vi "IFA300FrontPanel.vi"() -> ()   [LabVIEW 2011]
uses:
  subVIs/IFA300Command.ctl
  ADAM Client/Sub VIs/ADAM Controls/Remember_value_mode.ctl
  ADAM Client/Sub VIs/ADAM Controls/Update_scan_value.ctl
  Anemometry/Anemometry Sub Vis/Globals/Preference_global.vi
panel:
  in  "SquareWaveTest":bool
  out "CopytoChannels":string[](array[string])
  in  "ApplytoAll":bool
  in  "Cable Length":u8(slide)=1 max=1 step=1 scale=0.0..1.0
  in  "Overheat Setting":dbl(slide)=1.5 min=1.0 max=2.0 step=0.1 scale=1.0..2.0 scale format="%#.1f"
  in  "ModeArray":cluster{bool, "Enable":bool}[](array[cluster])
  in  "RunAll":bool caption="StopAll"
  in  "Reset IFA":bool
  out "Overheat (Running)":dbl format="%#.1f"
  in  "Port Name":string(combo)="COM4"
  out "Current Case":string="EndProgram"
  in  "EndProgram":bool
  in  "RunStandby":u8(knob) max=1 step=1 scale=0.0..1.0
  out "Standby":bool=TRUE
  out "Running":bool
  in  "Channel Selector":string(combo)="Channel 1"
  in  "Offset":dbl min=0.0 max=10.24 step=0.5 format="%#.2g"
  in  "Gain":string(combo)="1\r\n"
  in  "Low-Pass Filter":string(combo)="None"
  in  "High-Pass Filter":string(combo)="None"
  in  "High Power Bridge":u8(slide) max=1 step=1 scale=0.0..1.0
  in  "Probe Type Selector":u8(slide)=1 max=2 step=1 scale=0.0..2.0
  out "Temperature":dbl
  in  "StopAll":bool
  out "TimeColdResRead":string
  out "TimeColdResMeas":string
  out "TimeCableResRead":string
  out "TimeCableResMeas":string caption="Date/Time"
  in  "ReadColdRes":bool
  in  "ReadCableRes":bool
  in  "MeasColdRes":bool
  in  "MeasCableRes":bool
  out "Hot Resistance":dbl format="%#.2f"
  out "Probe Resistance":dbl format="%#.2f"
  out "Cable Resistance":dbl format="%#.2f"
  # "CH1"
  # "CH2"
  # "CH3"
  # "CH4"
  # "CH5"
  # "CH6"
  # "CH7"
  # "CH8"
  # "Running"
  # "Enabled"
  # "Disabled"
  # "Standby"
  # "Run"
  # "30m"
  # "5m"
  # "On"
  # "Off"
  # "Wire"
  # "Film"
  # "Non-Cylindrical"
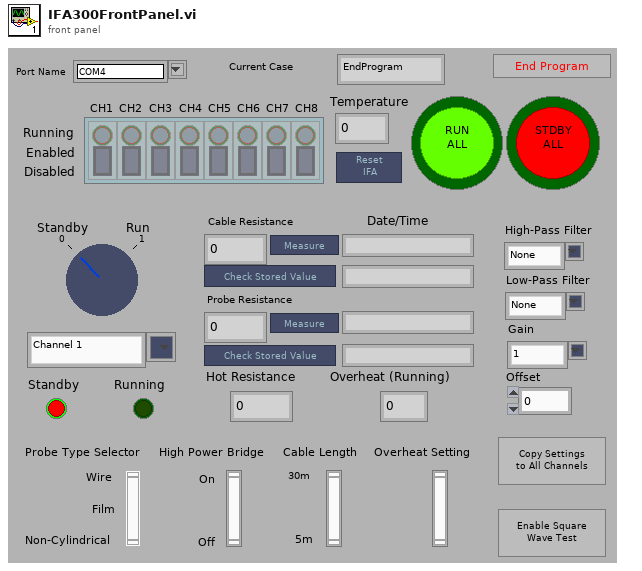
[diagram p1: front panel]
types:
  T1 = typedef "IFA300Command.ctl" = string
  T2 = typedef "Remember_value_mode.ctl" = enum16{"Read only", "Read and Write"}
  T3 = typedef "Update_scan_value.ctl" = cluster{"Channel Name":string, "New Value":dbl}
  T4 = cluster{"Running/Standby":string, "Enabled/Dissabled":string, "SecSince1904":string, "Date/TimeFileWritten":string}
  T5 = cluster{"Channel Selector":string, "RunAll":bool, "StopAll":bool, "EndProgram":bool, "MeasCableRes":bool, "ReadCableRes":bool, "MeasColdRes":bool, "ReadColdRes":bool, "Overheat Setting":dbl, "High-Pass Filter":string, "Low-Pass Filter":string, "Gain":string, "Offset":dbl, "RunStandby":u8, "Probe Type Selector":u8, "High Power Bridge":u8, "Cable Length":u8, "Reset IFA":bool, "ApplytoAll":bool, "SquareWaveTest":bool}
  T6 = cluster{"Channel Selector":bool, "RunAll":bool, "StopAll":bool, "EndProgram":bool, "MeasCableRes":bool, "ReadCableRes":bool, "MeasColdRes":bool, "ReadColdRes":bool, "Overheat Setting":bool, "High-Pass Filter":bool, "Low-Pass Filter":bool, "Gain":bool, "Offset":bool, "RunStandby":bool, "Probe Type Selector":bool, "High Power Bridge":bool, "Cable Length":bool, "Reset IFA":bool, "ApplytoAll":bool, "SquareWaveTest":bool}
  T7 = cluster{"Temperature":dbl, "Running":bool, "Standby":bool, "Cable Resistance":dbl, "Probe Resistance":dbl, "Hot Resistance":dbl, "Overheat (Running)":dbl, "Port Name":string, "TimeCableResMeas":string, "TimeCableResRead":string, "TimeColdResMeas":string, "TimeColdResRead":string}
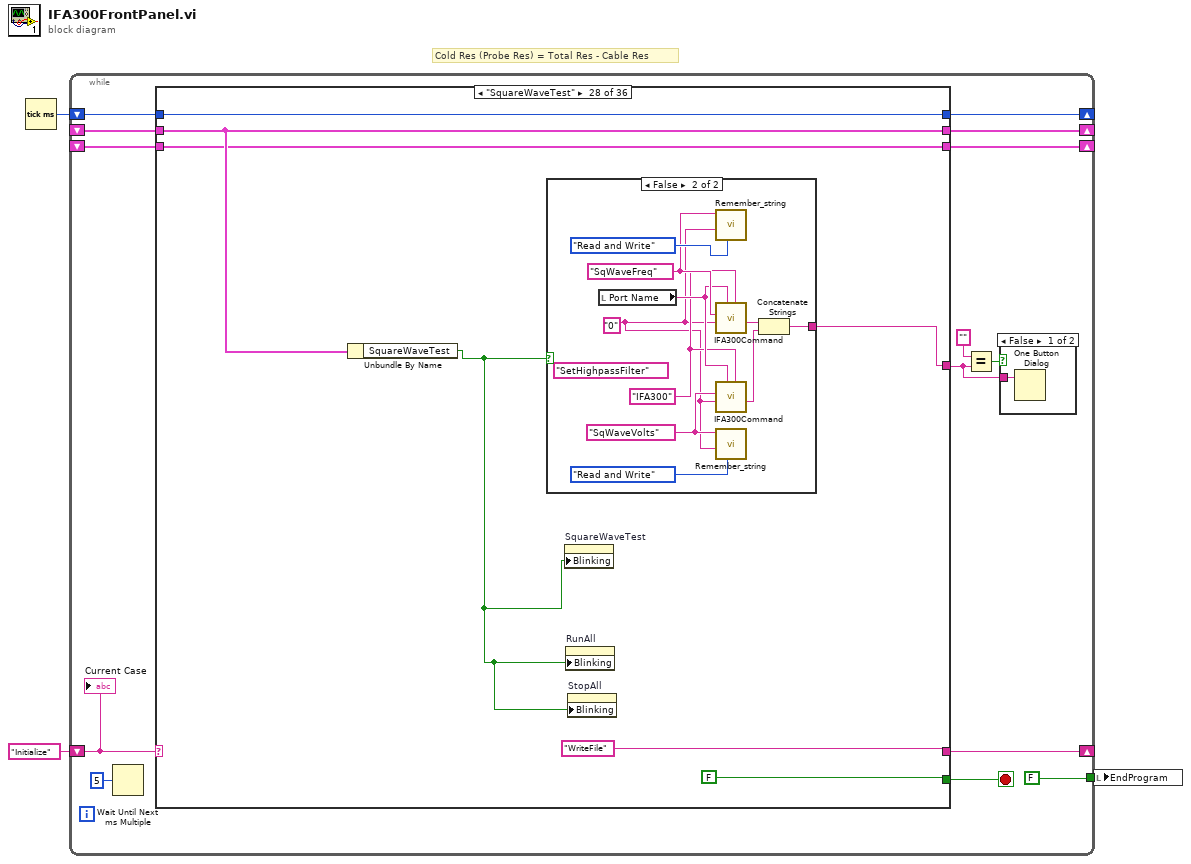
[diagram p0: block diagram]
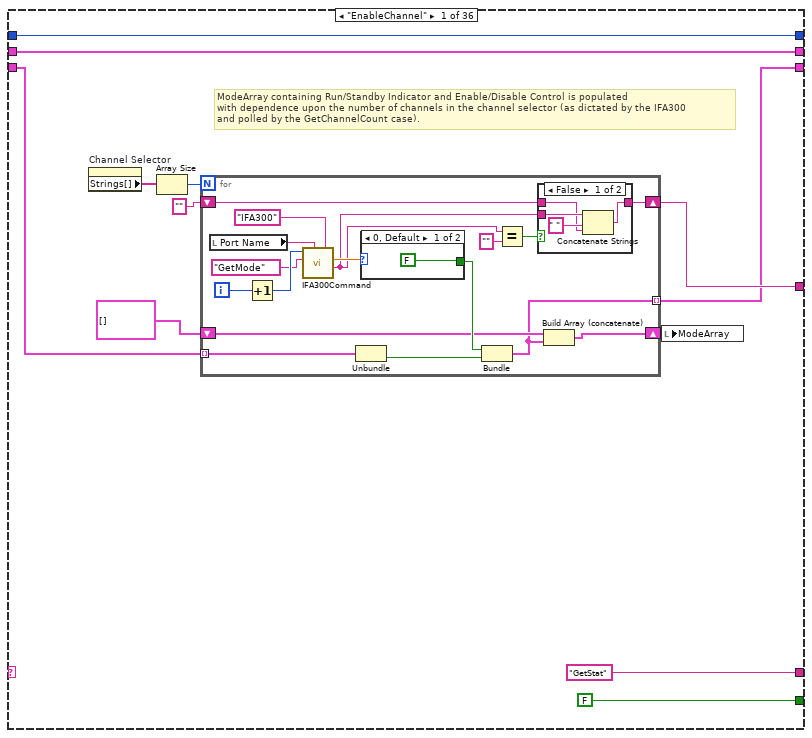
[diagram p3: hidden frame]
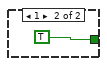
[diagram p5: hidden frame]
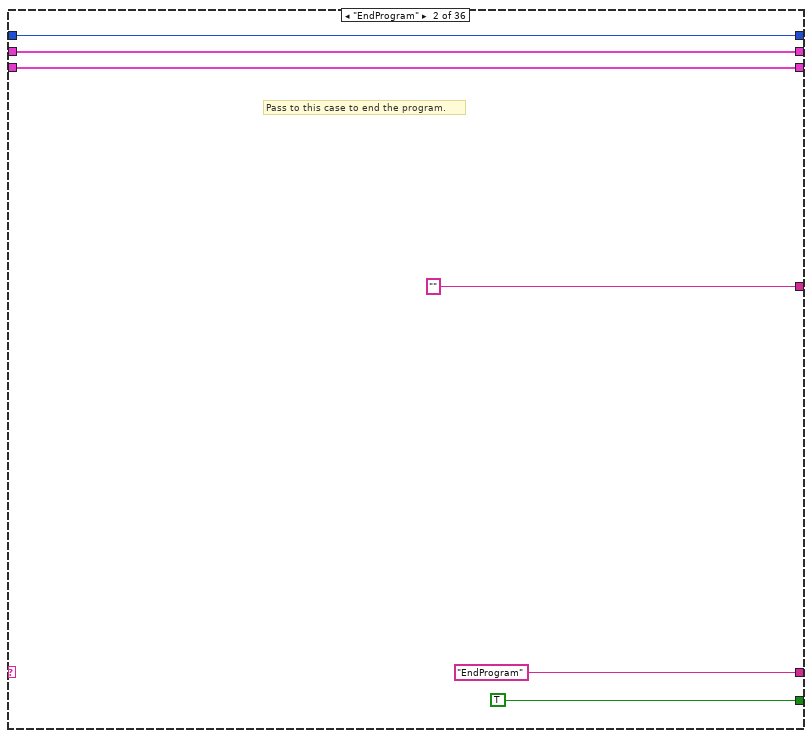
[diagram p6: hidden frame]
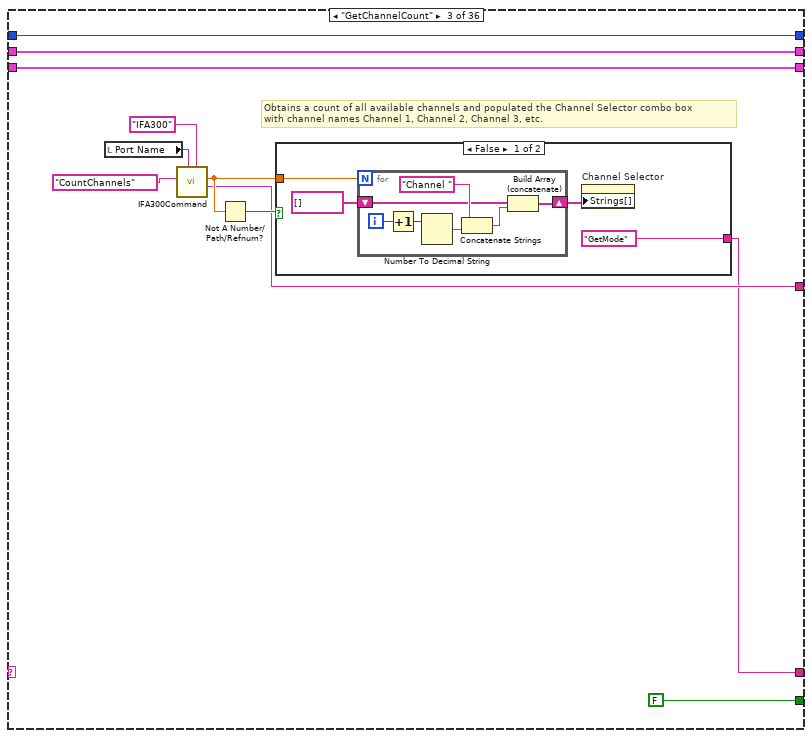
[diagram p7: hidden frame]
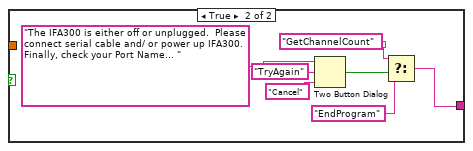
[diagram p8: hidden frame]
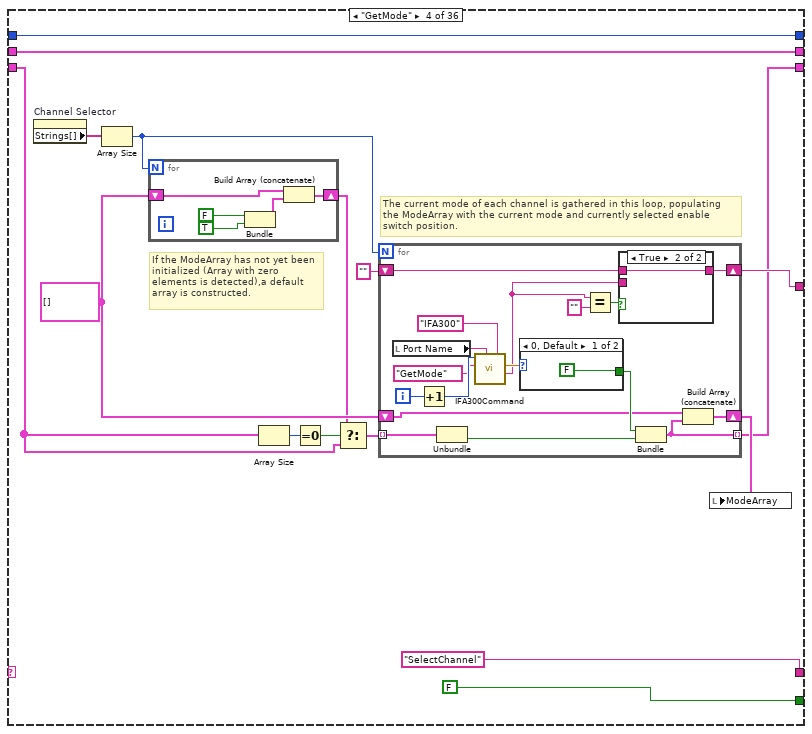
[diagram p9: hidden frame]
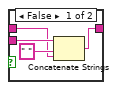
[diagram p10: hidden frame]
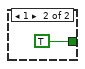
[diagram p11: hidden frame]
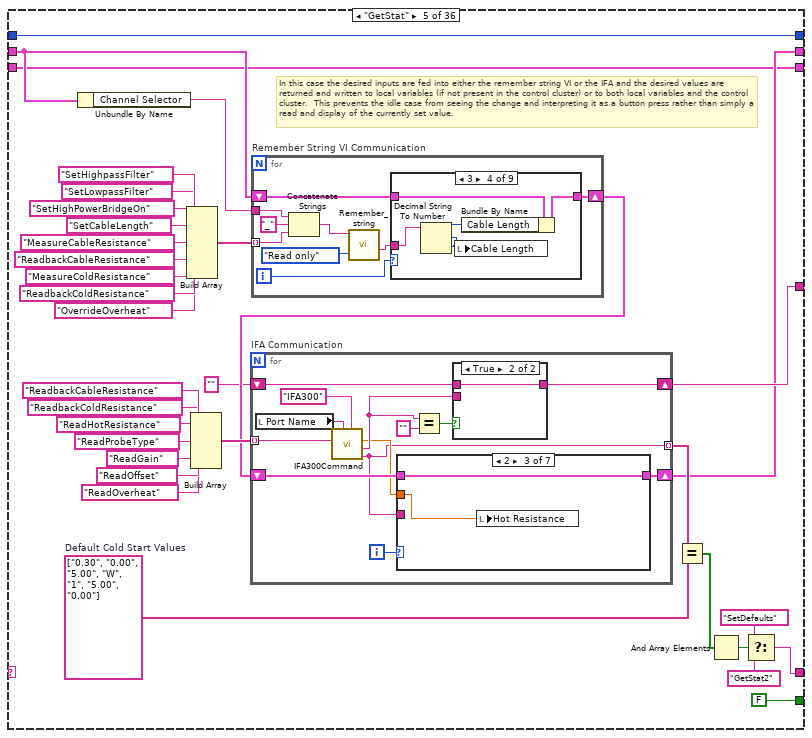
[diagram p12: hidden frame]
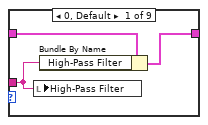
[diagram p13: hidden frame]
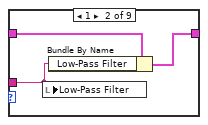
[diagram p14: hidden frame]
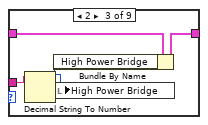
[diagram p15: hidden frame]
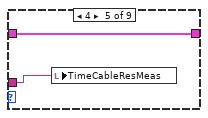
[diagram p16: hidden frame]
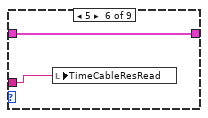
[diagram p17: hidden frame]
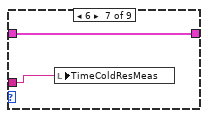
[diagram p18: hidden frame]
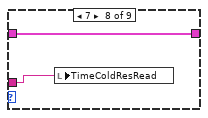
[diagram p19: hidden frame]
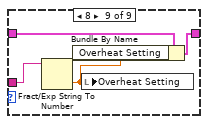
[diagram p20: hidden frame]
diagram:
  # "Cold Res (Probe Res) = Total Res - Cable Res"
  n1 = Tick Count (ms)() -> (millisecond timer value=w1:u32)
  n2 = while {
    shift-right: [w16] -> _
    shift-left: _ -> [w17]
    shift-right: [w14] -> _
    shift-left: "Initialize" -> [w12]
    tunnel: [FALSE ("EndProgram")] -> w2
    shift-right: [w6] -> _
    shift-left: w1 -> [w7]
    shift-right: [w5] -> _
    shift-left: _ -> [w4]
    stop <- w13 stop-if-true
    n3 = Wait Until Next ms Multiple(millisecond multiple=u32 5) -> ()  [unwired: 1 out]
    n4 = case shown="\"SquareWaveTest\"" w12 {
      tunnel: w17 -> [w28 w60 w64 w105 w145 w250 w290 w314 w371 _ w443 w464 w478 w486 w502 w533 w556 w573 w584 w598 w617 w624 w660 w685 w715 w795 w820 w835 w875 w905 w932 w967 w998 w1020 w1037 w1045]
      tunnel: [w28 w60 w64 w105 w137 w251 w290 w299 w375 w420 w443 w464 w478 w486 w502 w533 w556 w573 w584 w598 w617 w624 w660 w685 w716 w795 w820 w835 w875 w905 w932 w967 w998 w1020 w1037 w1071] -> w16
      tunnel: [FALSE ("EndProgram") TRUE ("EndProgram") FALSE ("EndProgram") FALSE ("EndProgram") FALSE ("EndProgram") FALSE ("EndProgram") FALSE ("EndProgram") FALSE ("EndProgram") FALSE ("EndProgram") FALSE ("EndProgram") FALSE ("EndProgram") FALSE ("EndProgram") FALSE ("EndProgram") TRUE ("EndProgram") FALSE ("EndProgram") FALSE ("EndProgram") FALSE ("EndProgram") FALSE ("EndProgram") FALSE ("EndProgram") FALSE ("EndProgram") FALSE ("EndProgram") FALSE ("EndProgram") FALSE ("EndProgram") FALSE ("EndProgram") FALSE ("EndProgram") FALSE ("EndProgram") FALSE ("EndProgram") FALSE ("EndProgram") FALSE ("EndProgram") FALSE ("EndProgram") FALSE ("EndProgram") FALSE ("EndProgram") FALSE ("EndProgram") FALSE ("EndProgram") FALSE ("EndProgram") FALSE ("EndProgram")] -> w13
      tunnel: ["GetStat" "EndProgram" w61 "SelectChannel" w155 "WriteFile" w272 w333 "SetProbeType" ("t") "GetChannelCount" "ReadCableRes" "ReadColdRes" "ReadTemperature" ("t") "NoMatch" w488 w523 "WriteFile" "WriteFile" "WriteFile" "Idle" ("t") "WriteFile" "GetMode" "GetStat" w668 "GetStat" ("t") w781 w802 "WriteFile" "ReadHotRes" w886 "GetMode" w956 w982 w1013 "GetMode" w1048] -> w14
      tunnel: [w21 "" ("Error Description") w65 w101 w161 w252 w289 "" ("Error Description") "" ("Error Description") "" ("x") w439 w462 w473 "" ("Error Description") w500 w522 w551 w565 w578 w600 w613 w622 w657 w680 w720 w793 w821 w831 w859 w901 w921 "" ("Error Description") w996 w1018 w1033 "" ("Error Description")] -> w8
      tunnel: w7 -> [w27 w56 w63 w99 w152 w259 w288 w335 w377 w402 w435 w458 _ w482 w498 w530 w549 w563 w577 w599 w612 w623 w656 w679 w717 w792 w812 w834 w863 w896 w926 w969 w995 w1017 w1031 w1080]
      tunnel: [w27 w56 w63 w99 w152 w259 w288 w335 w377 w402 w435 w458 w477 w482 w498 w530 w549 w563 w577 w599 w612 w623 w656 w679 w717 w792 w812 w834 w863 w896 w926 w969 w995 w1017 w1031 w1080] -> w6
      tunnel: [w19 w55 w62 w90 w136 w247 w277 w305 w376 "ModeArray" w426 w449 w472 w481 w487 w517 w548 w562 w576 w597 w606 w621 w655 w672 w714 w791 w806 w833 w858 w890 w914 w968 w994 w1016 w1030 w1077] -> w5
      tunnel: w4 -> [w20 w55 w62 w91 w136 w247 w277 w301 w376 _ w426 w449 w472 w481 w487 w517 w548 w562 w576 w597 w606 w621 w655 w672 w714 w791 w806 w833 w858 w890 w914 w968 w994 w1016 w1030 w1077]
      frame "EnableChannel" {
        # "ModeArray containing Run/Standby Indicator and Enable/Disable Control is populated\nwith dependence upon the number of channels in the channel selector (as dictated by the IFA300\nand polled by the GetChannelCount case)."
        n5 = property on="Channel Selector" class="CmbBox"() -> ("Strings[]"=w26:string[])  [unwired: 2 in, 2 out]
        n6 = Array Size(array=w26) -> (size(s)=w25:i32)
        n7 = for {
          N: w25 -> [_]
          shift-right: [w41] -> w21
          shift-left: "" -> [w40]
          shift-right: [w35] -> w22
          shift-left: cluster{bool, bool}[] [] -> [w34]
          tunnel: w20 -> [w33] mode=indexing
          tunnel: [w31] -> w19 mode=indexing
          i -> [w44]
          n8 = local read "Port Name"() -> (w46:string)
          n9 = Increment(x=w44) -> (x+1=w43:i32)
          n10 = call "IFA300Command.vi"("Channel Name"="IFA300", "Port Name"=w46, "IFACommand"=T1 "GetMode" ("IFA300Command"), "Address"=w43) -> ("Error Description"=w39:string, "Numeric Reply"=w45:dbl)  [unwired: 1 in, 4 out]
          n11 = Unbundle(w33) -> ("Enable"=w32:bool)  [unwired: 1 out]
          n12 = case shown="0, Default" w45 {
            tunnel: [FALSE TRUE] -> w36
            frame 0, Default {
            }
            frame 1 {
            }
          }
          n13 = Bundle(w36, "Enable"=w32) -> (w31:cluster{bool, "Enable":bool})  [unwired: 1 out]
          n14 = Equal?(x=w39, y="") -> (x = y?=w37:bool)
          n15 = case shown="False" w37 {
            tunnel: w39 -> [w50 _]
            tunnel: [w49 w52] -> w41
            tunnel: w40 -> [w48 w52]
            frame False {
              n16 = Concatenate Strings(w50, " " ("string"), w48) -> (w49:string)
            }
            frame True {
            }
          }
          n17 = Build Array (concatenate)(w34, w31) -> (w35:cluster{bool, "Enable":bool}[])
        }
        n18 = local write "ModeArray"(w22) -> ()
      }
      frame "EndProgram" {
        # "Pass to this case to end the program."
      }
      frame "GetChannelCount" {
        # "Obtains a count of all available channels and populated the Channel Selector combo box\nwith channel names Channel 1, Channel 2, Channel 3, etc."
        n19 = local read "Port Name"() -> (w69:string)
        n20 = call "IFA300Command.vi"("Channel Name"="IFA300", "Port Name"=w69, "IFACommand"=T1 "CountChannels" ("IFA300Command")) -> ("Error Description"=w65:string, "Numeric Reply"=w67:dbl)  [unwired: 2 in, 4 out]
        n21 = Not A Number/Path/Refnum?(number/path/refnum=w67) -> (NaN/Path/Refnum?=w66:bool)
        n22 = case shown="False" w66 {
          tunnel: w67 -> [w73 _]
          tunnel: ["GetMode" w84] -> w61
          frame False {
            n23 = for {
              N: w73 -> [_]
              shift-right: [w77] -> w74
              shift-left: string[] [] -> [w78]
              i -> [w81]
              n24 = Increment(x=w81) -> (x+1=w80:i32)
              n25 = Number To Decimal String(number=w80) -> (decimal integer string=w79:string)  [unwired: 1 out]
              n26 = Concatenate Strings("Channel ", w79) -> (w76:string)
              n27 = Build Array (concatenate)(w78, w76) -> (w77:string[])
            }
            n28 = property on="Channel Selector" class="CmbBox"("Strings[]"=w74) -> ()  [unwired: 2 in, 2 out]
          }
          frame True {
            n29 = Two Button Dialog(message="The IFA300 is either off or unplugged.  Please connect serial cable and/ or power up IFA300.  Finally, check your Port Name... ", 1:"Cancel" ("F button name (\"Cancel\")"), 2:"TryAgain" ("T button name (\"OK\")")) -> (T button?=w86:bool)
            n30 = Select(t="GetChannelCount", s=w86, f="EndProgram" ("t")) -> (s? t:f=w84:string)
          }
        }
      }
      frame "GetMode" {
        w93 = cluster{bool, bool}[] []
        # "The current mode of each channel is gathered in this loop, populating the ModeArray with the current mode and currently selected enable switch position."
        # "If the ModeArray has not yet been initialized (Array with zero elements is detected),a default array is constructed."
        n31 = property on="Channel Selector" class="CmbBox"() -> ("Strings[]"=w102:string[])  [unwired: 2 in, 2 out]
        n32 = Array Size(array=w102) -> (size(s)=w96:i32)
        n33 = for {
          N: w96 -> [_]
          shift-right: [w109] -> w92
          shift-left: w93 -> [w110]
          n34 = Bundle(FALSE, TRUE) -> (w108:cluster{bool, bool})  [unwired: 1 out]
          n35 = Build Array (concatenate)(w110, w108) -> (w109:cluster{bool, bool}[])
        }
        n36 = Array Size(array=w91) -> (size(s)=w97:i32)
        n37 = Equal To 0?(x=w97) -> (x = 0?=w95:bool)
        n38 = Select(t=w92, s=w95, f=w91) -> (s? t:f=w94:cluster{bool, "Enable":bool}[])
        n39 = for {
          N: w96 -> [_]
          shift-right: [w121] -> w101
          shift-left: "" -> [w120]
          shift-right: [w115] -> w98
          shift-left: w93 -> [w114]
          tunnel: w94 -> [w113] mode=indexing
          tunnel: [w111] -> w90 mode=indexing
          i -> [w124]
          n40 = local read "Port Name"() -> (w126:string)
          n41 = Increment(x=w124) -> (x+1=w123:i32)
          n42 = Unbundle(w113) -> ("Enable"=w112:bool)  [unwired: 1 out]
          n43 = call "IFA300Command.vi"("Channel Name"="IFA300", "Port Name"=w126, "IFACommand"=T1 "GetMode" ("IFA300Command"), "Address"=w123) -> ("Error Description"=w119:string, "Numeric Reply"=w125:dbl)  [unwired: 1 in, 4 out]
          n44 = case shown="0, Default" w125 {
            tunnel: [FALSE TRUE] -> w116
            frame 0, Default {
            }
            frame 1 {
            }
          }
          n45 = Equal?(x=w119, y="") -> (x = y?=w117:bool)
          n46 = case shown="True" w117 {
            tunnel: w119 -> [w130 _]
            tunnel: [w129 w132] -> w121
            tunnel: w120 -> [w128 w132]
            frame False {
              n47 = Concatenate Strings(w130, " " ("string"), w128) -> (w129:string)
            }
            frame True {
            }
          }
          n48 = Bundle(w116, "Enable"=w112) -> (w111:cluster{bool, "Enable":bool})  [unwired: 1 out]
          n49 = Build Array (concatenate)(w114, w111) -> (w115:cluster{bool, "Enable":bool}[])
        }
        n50 = local write "ModeArray"(w98) -> ()
      }
      frame "GetStat" {
        w159 = string[] ["0.30", "0.00", "5.00", "W", "1", "5.00", "0.00"]  # Default Cold Start Values
        # "In this case the desired inputs are fed into either the remember string VI or the IFA and the desired values are returned and written to local variables (if not present in the control cluster) or to both local variables and the control cluster.  This prevents the idle case from seeing the change and interpreting it as a button press rather than simply a read and display of the currently set value."
        n51 = Unbundle By Name(w145) -> ("Channel Selector"=w143:string)
        n52 = Build Array(T1 "SetHighpassFilter" ("IFA300Command"), T1 "SetLowpassFilter" ("IFA300Command"), T1 "SetHighPowerBridgeOn" ("IFA300Command"), T1 "SetCableLength" ("IFA300Command"), T1 "MeasureCableResistance" ("IFA300Command"), T1 "ReadbackCableResistance" ("IFA300Command"), T1 "MeasureColdResistance" ("IFA300Command"), T1 "ReadbackColdResistance" ("IFA300Command"), T1 "OverrideOverheat" ("element")) -> (w146:T1[])
        n53 = Build Array(T1 "ReadbackCableResistance" ("IFA300Command"), T1 "ReadbackColdResistance" ("IFA300Command"), T1 "ReadHotResistance" ("IFA300Command"), T1 "ReadProbeType" ("IFA300Command"), T1 "ReadGain" ("IFA300Command"), T1 "ReadOffset" ("IFA300Command"), T1 "ReadOverheat" ("IFA300Command")) -> (w160:T1[])
        n54 = for "Remember String VI Communication" {
          tunnel: w146 -> [w175] mode=indexing
          tunnel: w143 -> [w177]
          shift-right: [w169] -> w144
          shift-left: w145 -> [w170]
          i -> [w172]
          n55 = Concatenate Strings(w177, "_" ("string"), w175) -> (w174:string)
          n56 = call "Remember_string.vi"("Mode"=Remember_value_mode."Read only", "Ch name"=w174) -> ("Output Value"=w171:string)  [unwired: 2 in, 7 out]
          n57 = case shown="3" w172 {
            tunnel: w171 -> [w178 w181 w185 w189 w192 w194 w196 w198 w203]
            tunnel: w170 -> [w180 w183 w187 w191 w193 w195 w197 w199 w202]
            tunnel: [w179 w182 w186 w190 w193 w195 w197 w199 w201] -> w169
            frame 0, Default {
              n58 = local write "High-Pass Filter"(w178) -> ()
              n59 = Bundle By Name(cluster=w180, "High-Pass Filter"=w178) -> (w179:T5)
            }
            frame 1 {
              n60 = local write "Low-Pass Filter"(w181) -> ()
              n61 = Bundle By Name(cluster=w183, "Low-Pass Filter"=w181) -> (w182:T5)
            }
            frame 2 {
              n62 = Decimal String To Number(string=w185) -> (number=w184:i32)  [unwired: 3 out]
              n63 = Bundle By Name(cluster=w187, "High Power Bridge"=w184) -> (w186:T5)
              n64 = local write "High Power Bridge"(w184) -> ()
            }
            frame 3 {
              n65 = Decimal String To Number(string=w189) -> (number=w188:i32)  [unwired: 3 out]
              n66 = local write "Cable Length"(w188) -> ()
              n67 = Bundle By Name(cluster=w191, "Cable Length"=w188) -> (w190:T5)
            }
            frame 4 {
              n68 = local write "TimeCableResMeas"(w192) -> ()
            }
            frame 5 {
              n69 = local write "TimeCableResRead"(w194) -> ()
            }
            frame 6 {
              n70 = local write "TimeColdResMeas"(w196) -> ()
            }
            frame 7 {
              n71 = local write "TimeColdResRead"(w198) -> ()
            }
            frame 8 {
              n72 = Fract/Exp String To Number(string=w203) -> (number=w200:dbl)  [unwired: 4 out]
              n73 = Bundle By Name(cluster=w202, "Overheat Setting"=w200) -> (w201:T5)
              n74 = local write "Overheat Setting"(w200) -> ()
            }
          }
        }
        n75 = for "IFA Communication" {
          tunnel: w160 -> [w214] mode=indexing
          shift-right: [w211] -> w161
          shift-left: "" -> [w210]
          shift-right: [w205] -> w137
          shift-left: w144 -> [w207]
          tunnel: [w204] -> w151 mode=indexing
          i -> [w208]
          n76 = local read "Port Name"() -> (w215:string)
          n77 = call "IFA300Command.vi"("Channel Name"="IFA300", "Port Name"=w215, "IFACommand"=w214) -> ("String Reply"=w204:string, "Error Description"=w209:string, "Numeric Reply"=w206:dbl)  [unwired: 2 in, 3 out]
          n78 = case shown="2" w208 {
            tunnel: w207 -> [w218 w220 w222 w225 w232 w235 w236]
            tunnel: w204 -> [_ _ _ w224 w230 _ _]
            tunnel: w206 -> [w217 w219 w221 _ _ w233 w237]
            tunnel: [w218 w220 w222 w226 w231 w234 w236] -> w205
            frame 0, Default {
              n79 = local write "Cable Resistance"(w217) -> ()
            }
            frame 1 {
              n80 = local write "Probe Resistance"(w219) -> ()
            }
            frame 2 {
              n81 = local write "Hot Resistance"(w221) -> ()
            }
            frame 3 {
              n82 = case shown="\"F\", Default" w224 {
                tunnel: [u8 1 ("W/F/N Selector") u8 0 ("W/F/N Selector") u8 2 ("W/F/N Selector")] -> w223
                frame "F", Default {
                }
                frame "N" {
                }
                frame "W" {
                }
              }
              n83 = Bundle By Name(cluster=w225, "Probe Type Selector"=w223) -> (w226:T5)
              n84 = local write "Probe Type Selector"(w223) -> ()
            }
            frame 4 {
              n85 = local write "Gain"(w230) -> ()
              n86 = Bundle By Name(cluster=w232, "Gain"=w230) -> (w231:T5)
            }
            frame 5 {
              n87 = local write "Offset"(w233) -> ()
              n88 = Bundle By Name(cluster=w235, "Offset"=w233) -> (w234:T5)
            }
            frame 6 {
              n89 = local write "Overheat (Running)"(w237) -> ()
            }
          }
          n90 = Equal?(x=w209, y="") -> (x = y?=w213:bool)
          n91 = case shown="True" w213 {
            tunnel: w209 -> [w240 _]
            tunnel: [w239 w242] -> w211
            tunnel: w210 -> [w238 w242]
            frame False {
              n92 = Concatenate Strings(w240, " " ("string"), w238) -> (w239:string)
            }
            frame True {
            }
          }
        }
        n93 = Equal?(x=w151, y=w159) -> (x = y?=w158:bool[])
        n94 = And Array Elements(Boolean array=w158) -> (logical AND=w157:bool)
        n95 = Select(t="SetDefaults", s=w157, f="GetStat2") -> (s? t:f=w155:string)
      }
      frame "GetStat2" {
        # "This case controls the enabling/disabling of front panel controls.  The position of the enable/disable switch in the ModeArray is checked to determine current display.  Also, the current channel mode (Run/Standby) is polled and fed into a nesting case structure in the \"true\" case to further dictate the functions of the front panel controls while in run mode."
        n96 = Unbundle By Name(w250) -> ("Channel Selector"=w249:string)
        n97 = local read "Port Name"() -> (w257:string)
        n98 = String Subset(string=w249, offset (0)=8) -> (substring=w255:string)  [unwired: 1 out]
        n99 = Decimal String To Number(string=w255) -> (number=w245:i32)  [unwired: 3 out]
        n100 = call "IFA300Command.vi"("Channel Name"="IFA300", "Port Name"=w257, "IFACommand"=T1 "GetMode" ("IFA300Command"), "Address"=w245) -> ("String Reply"=w248:string, "Error Description"=w252:string, "Numeric Reply"=w253:dbl)  [unwired: 1 in, 3 out]
        n101 = Decrement(x=w245) -> (x-1=w244:i32)
        n102 = Index Array(array=w247, index=w244) -> (element=w246:cluster{bool, "Enable":bool})
        n103 = Unbundle(w246) -> ("Enable"=w243:bool)  [unwired: 1 out]
        n104 = local write "RunStandby"(w253) -> ()
        n105 = case shown="True" w243 {
          tunnel: w248 -> [_ w264]
          frame False {
            w262 = u8 2
            n106 = property on="Cable Resistance" class="DigNum (strict)"("Disabled"=w262) -> ()  [unwired: 2 in, 2 out]
            n107 = property on="Probe Resistance" class="DigNum (strict)"("Disabled"=w262) -> ()  [unwired: 2 in, 2 out]
            n108 = property on="RunStandby" class="Knob (strict)"("Disabled"=w262) -> ()  [unwired: 2 in, 2 out]
            n109 = property on="Running" class="Bool (strict)"("Disabled"=w262) -> ()  [unwired: 2 in, 2 out]
            n110 = property on="Standby" class="Bool (strict)"("Disabled"=w262) -> ()  [unwired: 2 in, 2 out]
            n111 = property on="MeasCableRes" class="Bool (strict)"("Disabled"=w262) -> ()  [unwired: 2 in, 2 out]
            n112 = property on="ReadCableRes" class="Bool (strict)"("Disabled"=w262) -> ()  [unwired: 2 in, 2 out]
            n113 = property on="MeasColdRes" class="Bool (strict)"("Disabled"=w262) -> ()  [unwired: 2 in, 2 out]
            n114 = property on="ReadColdRes" class="Bool (strict)"("Disabled"=w262) -> ()  [unwired: 2 in, 2 out]
            n115 = property on="Overheat Setting" class="Slide (strict)"("Disabled"=w262) -> ()  [unwired: 2 in, 2 out]
            n116 = property on="Overheat (Running)" class="DigNum (strict)"("Disabled"=w262) -> ()  [unwired: 2 in, 2 out]
            n117 = property on="Probe Type Selector" class="Slide (strict)"("Disabled"=w262) -> ()  [unwired: 2 in, 2 out]
            n118 = property on="High Power Bridge" class="Slide (strict)"("Disabled"=w262) -> ()  [unwired: 2 in, 2 out]
            n119 = property on="Cable Length" class="Slide (strict)"("Disabled"=w262) -> ()  [unwired: 2 in, 2 out]
            n120 = property on="TimeCableResMeas" class="Str"("Disabled"=w262) -> ()  [unwired: 2 in, 2 out]
            n121 = property on="TimeCableResRead" class="Str"("Disabled"=w262) -> ()  [unwired: 2 in, 2 out]
            n122 = property on="TimeColdResMeas" class="Str"("Disabled"=w262) -> ()  [unwired: 2 in, 2 out]
            n123 = property on="TimeColdResRead" class="Str"("Disabled"=w262) -> ()  [unwired: 2 in, 2 out]
            n124 = property on="Hot Resistance" class="DigNum (strict)"("Disabled"=w262) -> ()  [unwired: 2 in, 2 out]
            n125 = property on="High-Pass Filter" class="CmbBox"("Disabled"=w262) -> ()  [unwired: 2 in, 2 out]
            n126 = property on="Low-Pass Filter" class="CmbBox"("Disabled"=w262) -> ()  [unwired: 2 in, 2 out]
            n127 = property on="Gain" class="CmbBox"("Disabled"=w262) -> ()  [unwired: 2 in, 2 out]
            n128 = property on="Offset" class="DigNum (strict)"("Disabled"=w262) -> ()  [unwired: 2 in, 2 out]
          }
          frame True {
            w265 = u8 0
            n129 = case shown="\"1\"" w264 {
              tunnel: [u8 2 ("Disabled") u8 0 ("Disabled")] -> w263
              frame "1" {
                n130 = local write "Running"(TRUE) -> ()
                n131 = local write "Standby"(FALSE) -> ()
              }
              frame "0", Default {
                n132 = local write "Running"(FALSE) -> ()
                n133 = local write "Standby"(TRUE) -> ()
              }
            }
            n134 = property on="Cable Resistance" class="DigNum (strict)"("Disabled"=w265) -> ()  [unwired: 2 in, 2 out]
            n135 = property on="Probe Resistance" class="DigNum (strict)"("Disabled"=w265) -> ()  [unwired: 2 in, 2 out]
            n136 = property on="RunStandby" class="Knob (strict)"("Disabled"=w265) -> ()  [unwired: 2 in, 2 out]
            n137 = property on="Running" class="Bool (strict)"("Disabled"=w265) -> ()  [unwired: 2 in, 2 out]
            n138 = property on="Standby" class="Bool (strict)"("Disabled"=w265) -> ()  [unwired: 2 in, 2 out]
            n139 = property on="MeasCableRes" class="Bool (strict)"("Disabled"=w263) -> ()  [unwired: 2 in, 2 out]
            n140 = property on="ReadCableRes" class="Bool (strict)"("Disabled"=w265) -> ()  [unwired: 2 in, 2 out]
            n141 = property on="MeasColdRes" class="Bool (strict)"("Disabled"=w263) -> ()  [unwired: 2 in, 2 out]
            n142 = property on="ReadColdRes" class="Bool (strict)"("Disabled"=w265) -> ()  [unwired: 2 in, 2 out]
            n143 = property on="Overheat Setting" class="Slide (strict)"("Disabled"=w263) -> ()  [unwired: 2 in, 2 out]
            n144 = property on="Overheat (Running)" class="DigNum (strict)"("Disabled"=w265) -> ()  [unwired: 2 in, 2 out]
            n145 = property on="Probe Type Selector" class="Slide (strict)"("Disabled"=w263) -> ()  [unwired: 2 in, 2 out]
            n146 = property on="High Power Bridge" class="Slide (strict)"("Disabled"=w263) -> ()  [unwired: 2 in, 2 out]
            n147 = property on="Cable Length" class="Slide (strict)"("Disabled"=w263) -> ()  [unwired: 2 in, 2 out]
            n148 = property on="TimeCableResMeas" class="Str"("Disabled"=w265) -> ()  [unwired: 2 in, 2 out]
            n149 = property on="TimeCableResRead" class="Str"("Disabled"=w265) -> ()  [unwired: 2 in, 2 out]
            n150 = property on="TimeColdResMeas" class="Str"("Disabled"=w265) -> ()  [unwired: 2 in, 2 out]
            n151 = property on="TimeColdResRead" class="Str"("Disabled"=w265) -> ()  [unwired: 2 in, 2 out]
            n152 = property on="Hot Resistance" class="DigNum (strict)"("Disabled"=w265) -> ()  [unwired: 2 in, 2 out]
            n153 = property on="High-Pass Filter" class="CmbBox"("Disabled"=w265) -> ()  [unwired: 2 in, 2 out]
            n154 = property on="Low-Pass Filter" class="CmbBox"("Disabled"=w265) -> ()  [unwired: 2 in, 2 out]
            n155 = property on="Gain" class="CmbBox"("Disabled"=w265) -> ()  [unwired: 2 in, 2 out]
            n156 = property on="Offset" class="DigNum (strict)"("Disabled"=w265) -> ()  [unwired: 2 in, 2 out]
          }
        }
        n157 = Bundle By Name(cluster=w250, "RunStandby"=w253) -> (w251:T5)
      }
      frame "HighPowerBridge" {
        w278 = T1 "SetHighPowerBridgeOn" ("IFA300Command")
        # "Sets High Power Bridge and writes the value to Remember String VI due to lack of readback function with current hardware."
        n158 = Unbundle By Name(w290) -> ("Channel Selector"=w274:string, "High Power Bridge"=w279:u8)
        n159 = local read "ApplytoAll"() -> (w275:bool)
        n160 = case shown="True" w275 {
          tunnel: [w293 w295] -> w273
          tunnel: w274 -> [w293 _]
          tunnel: ["WriteFile" "SetCableLength"] -> w272
          frame False {
          }
          frame True {
            n161 = local read "CopytoChannels"() -> (w296:string[])
            n162 = Index Array(array=w296) -> (element=w295:string)  [unwired: 1 in]
          }
        }
        n163 = Number To Decimal String(number=w279) -> (decimal integer string=w276:string)  [unwired: 1 in]
        n164 = String Subset(string=w273, offset (0)=8) -> (substring=w284:string)  [unwired: 1 out]
        n165 = Decimal String To Number(string=w284) -> (number=w283:i32)  [unwired: 3 out]
        n166 = local read "Port Name"() -> (w286:string)
        n167 = Concatenate Strings(w273, "_" ("string"), w278) -> (w281:string)
        n168 = call "IFA300Command.vi"("Channel Name"="IFA300", "Port Name"=w286, "ValueToSet"=w276, "IFACommand"=w278, "Address"=w283) -> ("Error Description"=w289:string)  [unwired: 5 out]
        n169 = call "Remember_string.vi"("Mode"=Remember_value_mode."Read and Write", "Input Value"=w276, "Ch name"=w281) -> ()  [unwired: 1 in, 8 out]
      }
      frame "Idle" {
        n170 = local read "ModeArray"() -> (w305:cluster{bool, "Enable":bool}[])
        n171 = local read "Probe Type Selector"() -> (w319:u8)
        n172 = local read "High Power Bridge"() -> (w318:u8)
        n173 = local read "SquareWaveTest"() -> (w297:bool)
        n174 = local read "Channel Selector"() -> (w332:string)
        n175 = local read "Overheat Setting"() -> (w325:dbl)
        n176 = local read "High-Pass Filter"() -> (w324:string)
        n177 = local read "Low-Pass Filter"() -> (w323:string)
        n178 = local read "MeasCableRes"() -> (w329:bool)
        n179 = local read "ReadCableRes"() -> (w328:bool)
        n180 = local read "MeasColdRes"() -> (w327:bool)
        n181 = local read "ReadColdRes"() -> (w326:bool)
        n182 = local read "Cable Length"() -> (w317:u8)
        n183 = local read "EndProgram"() -> (w330:bool)
        n184 = local read "RunStandby"() -> (w320:u8)
        n185 = local read "ApplytoAll"() -> (w298:bool)
        n186 = local read "Reset IFA"() -> (w316:bool)
        n187 = local read "StopAll"() -> (w331:bool)
        n188 = local read "RunAll"() -> (w315:bool)
        n189 = local read "Offset"() -> (w321:dbl)
        n190 = Array Size(array=w305) -> (size(s)=w304:i32)
        n191 = Array Size(array=w301) -> (size(s)=w303:i32)
        n192 = local read "Gain"() -> (w322:string)
        n193 = Subtract(x=w304, y=w303) -> (x-y=w302:i32)
        n194 = for {
          N: w302 -> [_]
          shift-right: [w351] -> w300
          shift-left: w301 -> [w354]
          n195 = Bundle(FALSE, TRUE) -> (w352:cluster{bool, bool})  [unwired: 1 out]
          n196 = Build Array (concatenate)(w354, w352) -> (w351:cluster{bool, "Enable":bool}[])
        }
        n197 = Bundle By Name(cluster=w314, "Channel Selector"=w332, "RunAll"=w315, "StopAll"=w331, "EndProgram"=w330, "MeasCableRes"=w329, "ReadCableRes"=w328, "MeasColdRes"=w327, "ReadColdRes"=w326, "Overheat Setting"=w325, "High-Pass Filter"=w324, "Low-Pass Filter"=w323, "Gain"=w322, "Offset"=w321, "RunStandby"=w320, "Probe Type Selector"=w319, "High Power Bridge"=w318, "Cable Length"=w317, "Reset IFA"=w316, "ApplytoAll"=w298, "SquareWaveTest"=w297) -> (w299:T5)
        n198 = Equal?(x=w314, y=w299) -> (x = y?=w349:T6)
        n199 = Equal?(x=w300, y=w305) -> (x = y?=w313:cluster{bool, "Enable":bool}[])
        n200 = Tick Count (ms)() -> (millisecond timer value=w336:u32)
        n201 = Cluster To Array(cluster=w349) -> (array=w348:bool[])
        n202 = for {
          tunnel: w313 -> [w355] mode=indexing
          tunnel: [w356] -> w312 mode=indexing
          n203 = Unbundle(w355) -> (w358:bool, "Enable"=w357:bool)
          n204 = And(x=w358, y=w357) -> (x .and. y?=w356:bool)
        }
        n205 = Search 1D Array(1D array=w348, element=FALSE) -> (index of element=w341:i32)  [unwired: 1 out]
        n206 = Subtract(x=w336, y=w335) -> (x-y=w340:u32)
        n207 = Multiply(x=u32 30 ("y"), y=u32 1000) -> (x*y=w337:u32)
        n208 = Greater Or Equal To 0?(x=w341) -> (x >= 0?=w345:bool)
        n209 = Greater Or Equal?(x=w340, y=w337) -> (x >= y?=w334:bool)
        n210 = case shown="True" w345 {
          tunnel: string[] ["SelectChannel", "RunAll", "StandbyAll", "EndProgram", "MeasCableRes", "ReadCableRes", "MeasColdRes", "ReadColdRes", "SetOHRatio", "SetHighPassFilter", "SetLowPassFilter", "SetGain", "SetOffset", "SetMode", "SetProbeType", "HighPowerBridge", "SetCableLength", "ResetIFA", "ApplytoAll", "SquareWaveTest"] -> [_ w365]
          tunnel: [w359 w364] -> w308
          tunnel: w341 -> [_ w363]
          tunnel: w334 -> [w361 _]
          frame False {
            n211 = Select(t="MeasTemperature", s=w361, f="Idle") -> (s? t:f=w359:string)
          }
          frame True {
            n212 = Index Array(array=w365, index=w363) -> (element=w364:string)
          }
        }
        n213 = Search 1D Array(1D array=w312, element=FALSE) -> (index of element=w310:i32)  [unwired: 1 out]
        n214 = Greater Or Equal To 0?(x=w310) -> (x >= 0?=w309:bool)
        n215 = Select(t="EnableChannel", s=w309, f=w308) -> (s? t:f=w306:string)
        n216 = Select(t="WriteFile", s=w330, f=w306) -> (s? t:f=w333:string)
      }
      frame "ApplytoAll" {
        n217 = Unbundle By Name(w371) -> ("Channel Selector"=w370:string)
        n218 = local read "CopytoChannels"() -> (w368:string[])
        n219 = Empty Array?(array=w368) -> (empty?=w369:bool)
        n220 = case shown="True" w369 {
          tunnel: w370 -> [_ w380]
          frame False {
          }
          frame True {
            n221 = property on="Channel Selector" class="CmbBox"() -> ("Strings[]"=w381:string[])  [unwired: 2 in, 2 out]
            n222 = for {
              tunnel: w381 -> [w385] mode=indexing
              tunnel: w380 -> [w387]
              shift-right: [w383] -> w378
              shift-left: string[] [] -> [w382]
              n223 = Equal?(x=w387, y=w385) -> (x = y?=w386:bool)
              n224 = Build Array (concatenate)(w382, w385) -> (w384:string[])
              n225 = Select(t=w382, s=w386, f=w384) -> (s? t:f=w383:string[])
            }
            "CopytoChannels" <- w378
          }
        }
        n226 = Unbundle By Name(w371) -> ("ApplytoAll"=w367:bool)
        n227 = Not(x=w367) -> (.not. x?=w366:bool)
        n228 = Bundle By Name(cluster=w371, "ApplytoAll"=w366) -> (w375:T5)
      }
      frame "Initialize" {
        n229 = call "Serial_Port_Select.vi"("PortString"="IFA") -> ("SelectedPort"=w391:string, "PortList"=w392:string[])  [unwired: 8 in, 1 out]
        n230 = property on="Gain" class="CmbBox"("Strings[]"=string[] ["1", "2", "3", "4", "5", "6", "7", "8", "9", "10", "12", "14", "16", "18", "20", "25", "30", "40", "50", "60", "70", "80", "90", "100", "120", "140", "160", "180", "200", "250", "300", "350", "400", "500", "600", "700", "800", "900", "1000"] ("Strings []")) -> ()  [unwired: 2 in, 2 out]
        n231 = property on="Low-Pass Filter" class="CmbBox"("Strings[]"=string[] ["None", "10HZ", "100HZ", "300HZ", "1KHZ", "2KHZ", "5KHZ", "10KHZ", "20KHZ", "50KHZ", "100KHZ", "200KHZ", "500KHZ", "1MHZ"] ("Strings []")) -> ()  [unwired: 2 in, 2 out]
        n232 = property on="High-Pass Filter" class="CmbBox"("Strings[]"=string[] ["None", "10HZ", "1HZ", ".1HZ"] ("Strings []")) -> ()  [unwired: 2 in, 2 out]
        n233 = property on="Port Name" class="CmbBox"("Strings[]"=w392) -> ()  [unwired: 2 in, 2 out]
        n234 = call "IFA300Command.vi"("Channel Name"="IFA300", "Port Name"=w391, "IFACommand"=T1 "MeasureTemperature" ("IFA300Command")) -> ("String Reply"=w393:string)  [unwired: 2 in, 5 out]
        n235 = property on="Port Name" class="CmbBox"("Value"=w391) -> ()  [unwired: 2 in, 2 out]
        n236 = call "IFA300Command.vi"("Channel Name"="IFA300", "Port Name"=w391, "ValueToSet"=w393, "IFACommand"=T1 "ReadTemperature" ("IFA300Command")) -> ("Numeric Reply"=w396:dbl)  [unwired: 1 in, 5 out]
        n237 = local write "Temperature"(w396) -> ()
        n238 = Bundle("Channel Selector"="Channel Selector", "RunAll"="RunAll", "StopAll"="StopAll", "EndProgram"="EndProgram", "MeasCableRes"="MeasCableRes", "ReadCableRes"="ReadCableRes", "MeasColdRes"="MeasColdRes", "ReadColdRes"="ReadColdRes", "Overheat Setting"="Overheat Setting", "High-Pass Filter"="High-Pass Filter", "Low-Pass Filter"="Low-Pass Filter", "Gain"="Gain", "Offset"="Offset", "RunStandby"="RunStandby", "Probe Type Selector"="Probe Type Selector", "High Power Bridge"="High Power Bridge", "Cable Length"="Cable Length", "Reset IFA"="Reset IFA", "ApplytoAll"="ApplytoAll", "SquareWaveTest"="SquareWaveTest") -> (w420:T5)  [unwired: 1 out]
      }
      frame "MeasCableRes" {
        w428 = u32 5000 ("millisecond multiple")
        w432 = T1 "MeasureCableResistance" ("IFA300Command")
        n239 = Unbundle By Name(w443) -> ("Channel Selector"=w433:string)
        n240 = String Subset(string=w433, offset (0)=8) -> (substring=w441:string)  [unwired: 1 out]
        n241 = Decimal String To Number(string=w441) -> (number=w440:i32)  [unwired: 3 out]
        n242 = local read "Port Name"() -> (w444:string)
        n243 = Get Date/Time In Seconds() -> (seconds since 1Jan1904=w446:timestamp)
        n244 = call "ModalTimer.vi"("String"="Please wait while Cable Resistance is measured.", "MS to Wait"=w428) -> ()  [unwired: 10 out]
        n245 = Wait (ms)(milliseconds to wait=w428) -> (millisecond timer value=w436:u32)
        n246 = Format Date/Time String(seconds (now)=w446) -> (date/time string=w429:string)  [unwired: 2 out]
        n247 = Greater Than 0?(x=w436) -> (x > 0?=w438:bool)
        n248 = call "IFA300Command.vi"("Channel Name"="IFA300", "Port Name"=w444, "IFACommand"=w432, "Address"=w440) -> ("Error Description"=w439:string)  [unwired: 1 in, 5 out]
        n249 = local write "TimeCableResMeas"(w429) -> ()
        n250 = Not(x=w438) -> (.not. x?=w437:bool)
        n251 = local write "MeasCableRes"(w437) -> ()
        n252 = Concatenate Strings(w433, "_" ("string"), w432) -> (w431:string)
        n253 = call "Remember_string.vi"("Mode"=Remember_value_mode."Read and Write", "Input Value"=w429, "Ch name"=w431) -> ()  [unwired: 1 in, 8 out]
      }
      frame "MeasColdRes" {
        w450 = u32 5000 ("millisecond multiple")
        w454 = T1 "MeasureColdResistance" ("IFA300Command")
        n254 = Unbundle By Name(w464) -> ("Channel Selector"=w453:string)
        n255 = String Subset(string=w453, offset (0)=8) -> (substring=w466:string)  [unwired: 1 out]
        n256 = Decimal String To Number(string=w466) -> (number=w463:i32)  [unwired: 3 out]
        n257 = local read "Port Name"() -> (w467:string)
        n258 = Get Date/Time In Seconds() -> (seconds since 1Jan1904=w469:timestamp)
        n259 = Wait (ms)(milliseconds to wait=w450) -> (millisecond timer value=w459:u32)
        n260 = call "ModalTimer.vi"("String"="Please wait while Probe Resistance is measured.", "MS to Wait"=w450) -> ()  [unwired: 10 out]
        n261 = Format Date/Time String(seconds (now)=w469) -> (date/time string=w452:string)  [unwired: 2 out]
        n262 = Greater Than 0?(x=w459) -> (x > 0?=w461:bool)
        n263 = call "IFA300Command.vi"("Channel Name"="IFA300", "Port Name"=w467, "IFACommand"=w454, "Address"=w463) -> ("Error Description"=w462:string)  [unwired: 1 in, 5 out]
        n264 = local write "TimeColdResMeas"(w452) -> ()
        n265 = Not(x=w461) -> (.not. x?=w460:bool)
        n266 = local write "MeasColdRes"(w460) -> ()
        n267 = Concatenate Strings(w453, "_" ("string"), w454) -> (w456:string)
        n268 = call "Remember_string.vi"("Mode"=Remember_value_mode."Read and Write", "Input Value"=w452, "Ch name"=w456) -> ()  [unwired: 1 in, 8 out]
      }
      frame "MeasTemperature" {
        n269 = local read "Port Name"() -> (w475:string)
        n270 = call "IFA300Command.vi"("Channel Name"="IFA300", "Port Name"=w475, "IFACommand"=T1 "MeasureTemperature" ("IFA300Command")) -> ("Error Description"=w473:string)  [unwired: 2 in, 5 out]
        n271 = Tick Count (ms)() -> (millisecond timer value=w477:u32)
      }
      frame "NoMatch", Default {
      }
      frame "ReadCableRes" {
        w494 = T1 "ReadbackCableResistance" ("IFA300Command")
        n272 = Unbundle By Name(w502) -> ("Channel Selector"=w493:string)
        n273 = String Subset(string=w493, offset (0)=8) -> (substring=w503:string)  [unwired: 1 out]
        n274 = local read "Port Name"() -> (w505:string)
        n275 = Get Date/Time In Seconds() -> (seconds since 1Jan1904=w507:timestamp)
        n276 = Decimal String To Number(string=w503) -> (number=w501:i32)  [unwired: 3 out]
        n277 = Format Date/Time String(seconds (now)=w507) -> (date/time string=w492:string)  [unwired: 2 out]
        n278 = local write "TimeCableResRead"(w492) -> ()
        n279 = call "IFA300Command.vi"("Channel Name"="IFA300", "Port Name"=w505, "IFACommand"=w494, "Address"=w501) -> ("Error Description"=w500:string, "Numeric Reply"=w489:dbl)  [unwired: 1 in, 4 out]
        n280 = local write "Cable Resistance"(w489) -> ()
        n281 = Concatenate Strings(w493, "_" ("string"), w494) -> (w496:string)
        n282 = Greater?(x=w489, y=2.5) -> (0:w490:bool)
        n283 = call "Remember_string.vi"("Mode"=Remember_value_mode."Read and Write", "Input Value"=w492, "Ch name"=w496) -> ()  [unwired: 1 in, 8 out]
        n284 = case shown="True" w490 {
          tunnel: ["WriteFile" w511] -> w488
          frame False {
          }
          frame True {
            n285 = Two Button Dialog(message="Erroneous Cable Resistance value measured, please check connections and ensure SHORTING PROBE is inserted.", 1:"I Didn't Want to Do That" ("F button name (\"Cancel\")"), 2:"I Fixed It, Try Again" ("T button name (\"OK\")")) -> (T button?=w513:bool)
            n286 = Select(t="MeasCableRes", s=w513, f="Idle") -> (s? t:f=w511:string)
          }
        }
        n287 = local write "ReadCableRes"(FALSE ("ReadCableRes")) -> ()
      }
      frame "ReadColdRes" {
        w525 = T1 "ReadbackColdResistance" ("IFA300Command")
        n288 = Get Date/Time In Seconds() -> (seconds since 1Jan1904=w538:timestamp)
        n289 = Unbundle By Name(w533) -> ("Channel Selector"=w526:string)
        n290 = Format Date/Time String(seconds (now)=w538) -> (date/time string=w524:string)  [unwired: 2 out]
        n291 = local write "TimeColdResRead"(w524) -> ()
        n292 = Concatenate Strings(w526, "_" ("string"), w525) -> (w528:string)
        n293 = String Subset(string=w526, offset (0)=8) -> (substring=w535:string)  [unwired: 1 out]
        n294 = call "Remember_string.vi"("Mode"=Remember_value_mode."Read and Write", "Input Value"=w524, "Ch name"=w528) -> ()  [unwired: 1 in, 8 out]
        n295 = Decimal String To Number(string=w535) -> (number=w532:i32)  [unwired: 3 out]
        n296 = local read "Port Name"() -> (w536:string)
        n297 = call "IFA300Command.vi"("Channel Name"="IFA300", "Port Name"=w536, "IFACommand"=w525, "Address"=w532) -> ("Error Description"=w522:string, "Numeric Reply"=w519:dbl)  [unwired: 1 in, 4 out]
        n298 = local write "Probe Resistance"(w519) -> ()
        n299 = In Range and Coerce(upper limit=10.0 ("y"), x=w519, lower limit=2.0 ("y")) -> (In Range?=w518:bool)  [unwired: 1 out]
        n300 = case shown="False" w518 {
          tunnel: [w540 "SetHotRes"] -> w523
          frame False {
            n301 = Two Button Dialog(message="Erroneous Probe Resistance value measured, please check connections and ensure HOTFILM PROBE is inserted.", 1:"I Didn't Want to Do That" ("F button name (\"Cancel\")"), 2:"I Fixed It, Try Again" ("T button name (\"OK\")")) -> (T button?=w543:bool)
            n302 = Select(t="MeasColdRes", s=w543, f="WriteFile") -> (s? t:f=w540:string)
          }
          frame True {
          }
        }
        n303 = local write "ReadColdRes"(FALSE ("ReadColdRes")) -> ()
      }
      frame "ReadGain" {
        n304 = Unbundle By Name(w556) -> ("Channel Selector"=w555:string)
        n305 = String Subset(string=w555, offset (0)=8) -> (substring=w553:string)  [unwired: 1 out]
        n306 = Decimal String To Number(string=w553) -> (number=w552:i32)  [unwired: 3 out]
        n307 = local read "Port Name"() -> (w558:string)
        n308 = call "IFA300Command.vi"("Channel Name"="IFA300", "Port Name"=w558, "IFACommand"=T1 "ReadGain" ("IFA300Command"), "Address"=w552) -> ("String Reply"=w550:string, "Error Description"=w551:string)  [unwired: 1 in, 4 out]
        n309 = local write "Gain"(w550) -> ()
      }
      frame "ReadHotRes" {
        n310 = Unbundle By Name(w573) -> ("Channel Selector"=w567:string)
        n311 = String Subset(string=w567, offset (0)=8) -> (substring=w568:string)  [unwired: 1 out]
        n312 = Decimal String To Number(string=w568) -> (number=w566:i32)  [unwired: 3 out]
        n313 = local read "Port Name"() -> (w572:string)
        n314 = call "IFA300Command.vi"("Channel Name"="IFA300", "Port Name"=w572, "IFACommand"=T1 "ReadHotResistance" ("IFA300Command"), "Address"=w566) -> ("Error Description"=w565:string, "Numeric Reply"=w564:dbl)  [unwired: 1 in, 4 out]
        n315 = local write "Hot Resistance"(w564) -> ()
      }
      frame "ReadOffset" {
        n316 = Unbundle By Name(w584) -> ("Channel Selector"=w581:string)
        n317 = String Subset(string=w581, offset (0)=8) -> (substring=w582:string)  [unwired: 1 out]
        n318 = Decimal String To Number(string=w582) -> (number=w580:i32)  [unwired: 3 out]
        n319 = local read "Port Name"() -> (w586:string)
        n320 = call "IFA300Command.vi"("Channel Name"="IFA300", "Port Name"=w586, "IFACommand"=T1 "ReadOffset" ("IFA300Command"), "Address"=w580) -> ("Error Description"=w578:string, "Numeric Reply"=w579:dbl)  [unwired: 1 in, 4 out]
        n321 = local write "Offset"(w579) -> ()
      }
      frame "ReadTemperature" {
        n322 = global read "Preference_global.vi" "Rig Setup"() -> (w592:string)
        n323 = local read "Port Name"() -> (w602:string)
        n324 = call "IFA300Command.vi"("Channel Name"="IFA300", "Port Name"=w602, "IFACommand"=T1 "ReadTemperature" ("IFA300Command")) -> ("Error Description"=w600:string, "Numeric Reply"=w593:dbl)  [unwired: 2 in, 4 out]
        n325 = local write "Temperature"(w593) -> ()
        n326 = Concatenate Strings(w592, ":IFA300:Temperature" ("Channel Name")) -> (w590:string)
        n327 = Bundle By Name(cluster=T3 {"Channel Name"="", "New Value"=0.0} ("Update Scan Value Cluster"), "Channel Name"=w590, "New Value"=w593) -> (w595:T3)
        n328 = Build Array(w595) -> (w594:T3[])
        n329 = call "Update_Current_Value_client.vi"("Update array in"=w594) -> ()  [unwired: 1 in]
      }
      frame "ResetIFA" {
        w607 = u32 5000 ("millisecond multiple")
        n330 = local read "Port Name"() -> (w615:string)
        n331 = call "IFA300Command.vi"("Channel Name"="IFA300", "Port Name"=w615, "IFACommand"=T1 "Reset" ("IFA300Command")) -> ("Error Description"=w613:string)  [unwired: 2 in, 5 out]
        n332 = Wait (ms)(milliseconds to wait=w607) -> (millisecond timer value=w610:u32)
        n333 = call "ModalTimer.vi"("String"="Please wait while IFA300 is reset.", "MS to Wait"=w607) -> ()  [unwired: 10 out]
        n334 = Greater Than 0?(x=w610) -> (x > 0?=w611:bool)
        n335 = Not(x=w611) -> (.not. x?=w609:bool)
        n336 = local write "Reset IFA"(w609) -> ()
      }
      frame "RunAll" {
        n337 = for {
          tunnel: [w630] -> w622
          tunnel: w621 -> [w629] mode=indexing
          i -> [w627]
          n338 = Unbundle(w629) -> ("Enable"=w628:bool)  [unwired: 1 out]
          n339 = case shown="True" w628 {
            tunnel: ["" ("Error Description") w642] -> w630
            tunnel: w627 -> [_ w635]
            frame False {
            }
            frame True {
              n340 = Increment(x=w635) -> (x+1=w634:i32)
              n341 = local read "Port Name"() -> (w638:string)
              n342 = call "IFA300Command.vi"("Channel Name"="IFA300", "Port Name"=w638, "IFACommand"=T1 "RunMode" ("IFA300Command"), "Address"=w634) -> ("Error Description"=w643:string)  [unwired: 1 in, 5 out]
              n343 = Equal?(x=w643, y="") -> (x = y?=w633:bool)
              n344 = local read "ModeArray"() -> (w641:cluster{bool, "Enable":bool}[])
              n345 = local write "Running"(w633) -> ()
              n346 = Not(x=w633) -> (.not. x?=w632:bool)
              n347 = case shown="False" w633 {
                tunnel: w643 -> [w646 w654]
                tunnel: ["" ("Error Description") w654] -> w642
                tunnel: w634 -> [w649 _]
                frame False {
                  n348 = Number To Decimal String(number=w649) -> (decimal integer string=w648:string)  [unwired: 1 out]
                  n349 = Concatenate Strings("Unable to set Channel ", w648, " to Run mode.  Check Cable Res and Cold Res values and retry." ("string"), "\n\n" ("string"), "Error Code: " ("string"), w646) -> (w650:string)
                  n350 = One Button Dialog(message=w650) -> ()  [unwired: 2 out]
                }
                frame True {
                }
              }
              n351 = Bundle(w633, w633) -> (w639:cluster{bool, bool})  [unwired: 1 out]
              n352 = local write "Standby"(w632) -> ()
              n353 = Replace Array Subset(array=w641, new element=w639, index=w635) -> (w640:cluster{bool, "Enable":bool}[])
              n354 = local write "ModeArray"(w640) -> ()
            }
          }
        }
        n355 = local write "RunAll"(FALSE ("RunAll")) -> ()
      }
      frame "SelectChannel" {
        n356 = Unbundle By Name(w660) -> ("Channel Selector"=w659:string)
        n357 = String Subset(string=w659, offset (0)=8) -> (substring=w661:string)  [unwired: 1 out]
        n358 = Decimal String To Number(string=w661) -> (number=w658:i32)  [unwired: 3 out]
        n359 = local read "Port Name"() -> (w664:string)
        n360 = call "IFA300Command.vi"("Channel Name"="IFA300", "Port Name"=w664, "IFACommand"=T1 "SelectChannel" ("IFA300Command"), "Address"=w658) -> ("Error Description"=w657:string)  [unwired: 1 in, 5 out]
      }
      frame "SetCableLength" {
        w674 = T1 "SetCableLength" ("IFA300Command")
        n361 = local read "ApplytoAll"() -> (w671:bool)
        n362 = Unbundle By Name(w685) -> ("Channel Selector"=w670:string, "Cable Length"=w673:u8)
        n363 = case shown="True" w671 {
          tunnel: [w690 w692] -> w669
          tunnel: w670 -> [w690 _]
          tunnel: ["WriteFile" "SetOHRatio"] -> w668
          frame False {
          }
          frame True {
            n364 = local read "CopytoChannels"() -> (w693:string[])
            n365 = Index Array(array=w693) -> (element=w692:string)  [unwired: 1 in]
          }
        }
        n366 = case shown="0, Default" w673 {
          tunnel: ["0" "20"] -> w684
          frame 0, Default {
          }
          frame 1 {
          }
        }
        n367 = Concatenate Strings(w669, "_" ("string"), w674) -> (w677:string)
        n368 = Number To Decimal String(number=w673) -> (decimal integer string=w675:string)  [unwired: 1 out]
        n369 = call "Remember_string.vi"("Mode"=Remember_value_mode."Read and Write", "Input Value"=w675, "Ch name"=w677) -> ()  [unwired: 1 in, 8 out]
        n370 = String Subset(string=w669, offset (0)=8) -> (substring=w682:string)  [unwired: 1 out]
        n371 = local read "Port Name"() -> (w686:string)
        n372 = Decimal String To Number(string=w682) -> (number=w681:i32)  [unwired: 3 out]
        n373 = call "IFA300Command.vi"("Channel Name"="IFA300", "Port Name"=w686, "ValueToSet"=w684, "IFACommand"=w674, "Address"=w681) -> ("Error Description"=w680:string)  [unwired: 5 out]
      }
      frame "SetDefaults" {
        w704 = string[] ["Insert Shorting Probe", "Not Yet Read", "Insert Hotfilm Probe", "Not Yet Read", "1.5"]  # Default Values
        w709 = string[] ["F", "1", "0.00", "BVSC", "BVSC", "0", "20"]  # Default IFA300 Setting Values
        n374 = Unbundle By Name(w715) -> ("Channel Selector"=w698:string)
        n375 = Build Array(T1 "SetProbeType" ("IFA300Command"), T1 "SetGain" ("IFA300Command"), T1 "SetOffset" ("IFA300Command"), T1 "SetHighpassFilter" ("IFA300Command"), T1 "SetLowpassFilter" ("IFA300Command"), T1 "SetHighPowerBridgeOn" ("IFA300Command"), T1 "SetCableLength" ("IFA300Command")) -> (w710:T1[])
        n376 = Build Array(T1 "MeasureCableResistance" ("IFA300Command"), T1 "ReadbackCableResistance" ("IFA300Command"), T1 "MeasureColdResistance" ("IFA300Command"), T1 "ReadbackColdResistance" ("IFA300Command"), T1 "OverrideOverheat" ("element")) -> (w699:T1[])
        n377 = for {
          tunnel: w704 -> [w725] mode=indexing
          tunnel: w698 -> [w724]
          tunnel: w699 -> [w721] mode=indexing
          n378 = Concatenate Strings(w724, "_" ("string"), w721) -> (w723:string)
          n379 = call "Remember_string.vi"("Mode"=Remember_value_mode."Read and Write", "Input Value"=w725, "Ch name"=w723) -> ()  [unwired: 1 in, 8 out]
        }
        n380 = for {
          tunnel: w710 -> [w730] mode=indexing
          shift-right: [w734] -> w720
          shift-left: "" -> [w733]
          tunnel: w709 -> [w731] mode=indexing
          shift-right: [w728] -> w716
          shift-left: w715 -> [w729]
          tunnel: w698 -> [w727]
          n381 = local read "Port Name"() -> (w737:string)
          n382 = case shown="\"SetCableLength\"" w730 {
            selector: w730 -> [_ _ _ w746 w751 w760 w770]
            tunnel: w729 -> [w739 w740 w741 w749 w756 w766 w775]
            tunnel: [w739 w740 w741 w748 w757 w765 w774] -> w728
            tunnel: w727 -> [_ _ _ w747 w752 w761 w769]
            frame "SetProbeType", Default {
            }
            frame "SetGain" {
            }
            frame "SetOffset" {
            }
            frame "SetHighpassFilter" {
              w743 = "None"
              n383 = Concatenate Strings(w747, "_" ("string"), w746) -> (w744:string)
              n384 = local write "High-Pass Filter"(w743) -> ()
              n385 = Bundle By Name(cluster=w749, "High-Pass Filter"=w743) -> (w748:T5)
              n386 = call "Remember_string.vi"("Mode"=Remember_value_mode."Read and Write", "Input Value"=w743, "Ch name"=w744) -> ()  [unwired: 1 in, 8 out]
            }
            frame "SetLowpassFilter" {
              w750 = "None"
              n387 = Concatenate Strings(w752, "_" ("string"), w751) -> (w754:string)
              n388 = local write "Low-Pass Filter"(w750) -> ()
              n389 = Bundle By Name(cluster=w756, "Low-Pass Filter"=w750) -> (w757:T5)
              n390 = call "Remember_string.vi"("Mode"=Remember_value_mode."Read and Write", "Input Value"=w750, "Ch name"=w754) -> ()  [unwired: 1 in, 8 out]
            }
            frame "SetHighPowerBridgeOn" {
              w759 = u8 0 ("High Power Bridge")
              n391 = local write "High Power Bridge"(w759) -> ()
              n392 = Bundle By Name(cluster=w766, "High Power Bridge"=w759) -> (w765:T5)
              n393 = Number To Decimal String(number=w759) -> (decimal integer string=w758:string)  [unwired: 1 out]
              n394 = Concatenate Strings(w761, "_" ("string"), w760) -> (w763:string)
              n395 = call "Remember_string.vi"("Mode"=Remember_value_mode."Read and Write", "Input Value"=w758, "Ch name"=w763) -> ()  [unwired: 1 in, 8 out]
            }
            frame "SetCableLength" {
              w767 = u8 1 ("High Power Bridge")
              n396 = Number To Decimal String(number=w767) -> (decimal integer string=w768:string)  [unwired: 1 out]
              n397 = local write "Cable Length"(w767) -> ()
              n398 = Concatenate Strings(w769, "_" ("string"), w770) -> (w772:string)
              n399 = Bundle By Name(cluster=w775, "Cable Length"=w767) -> (w774:T5)
              n400 = call "Remember_string.vi"("Mode"=Remember_value_mode."Read and Write", "Input Value"=w768, "Ch name"=w772) -> ()  [unwired: 1 in, 8 out]
            }
          }
          n401 = call "IFA300Command.vi"("Channel Name"="IFA300", "Port Name"=w737, "ValueToSet"=w731, "IFACommand"=w730) -> ("Error Description"=w732:string)  [unwired: 1 in, 5 out]
          n402 = Equal?(x=w732, y="") -> (x = y?=w736:bool)
          n403 = case shown="True" w736 {
            tunnel: w732 -> [w778 _]
            tunnel: [w777 w780] -> w734
            tunnel: w733 -> [w776 w780]
            frame False {
              n404 = Concatenate Strings(w778, " " ("string"), w776) -> (w777:string)
            }
            frame True {
            }
          }
        }
      }
      frame "SetGain" {
        n405 = Unbundle By Name(w795) -> ("Channel Selector"=w783:string, "Gain"=w794:string)
        n406 = local read "ApplytoAll"() -> (w784:bool)
        n407 = case shown="True" w784 {
          tunnel: [w798 w800] -> w782
          tunnel: w783 -> [w798 _]
          tunnel: ["ReadGain" "SetOffset"] -> w781
          frame False {
          }
          frame True {
            n408 = local read "CopytoChannels"() -> (w801:string[])
            n409 = Index Array(array=w801) -> (element=w800:string)  [unwired: 1 in]
          }
        }
        n410 = String Subset(string=w782, offset (0)=8) -> (substring=w786:string)  [unwired: 1 out]
        n411 = Decimal String To Number(string=w786) -> (number=w785:i32)  [unwired: 3 out]
        n412 = local read "Port Name"() -> (w789:string)
        n413 = call "IFA300Command.vi"("Channel Name"="IFA300", "Port Name"=w789, "ValueToSet"=w794, "IFACommand"=T1 "SetGain" ("IFA300Command"), "Address"=w785) -> ("Error Description"=w793:string)  [unwired: 5 out]
      }
      frame "SetHighPassFilter" {
        w810 = T1 "SetHighpassFilter" ("IFA300Command")
        n414 = local read "ApplytoAll"() -> (w805:bool)
        n415 = Unbundle By Name(w820) -> ("Channel Selector"=w804:string, "High-Pass Filter"=w807:string)
        n416 = case shown="True" w805 {
          tunnel: [w826 w828] -> w803
          tunnel: w804 -> [w826 _]
          tunnel: ["WriteFile" "SetLowPassFilter"] -> w802
          frame False {
          }
          frame True {
            n417 = local read "CopytoChannels"() -> (w829:string[])
            n418 = Index Array(array=w829) -> (element=w828:string)  [unwired: 1 in]
          }
        }
        n419 = String Subset(string=w803, offset (0)=8) -> (substring=w818:string)  [unwired: 1 out]
        n420 = Equal?(x=w807, y="None") -> (x = y?=w815:bool)
        n421 = Concatenate Strings(w803, "_" ("string"), w810) -> (w809:string)
        n422 = Decimal String To Number(string=w818) -> (number=w817:i32)  [unwired: 3 out]
        n423 = Select(t="BVSC", s=w815, f=w807) -> (s? t:f=w814:string)
        n424 = call "Remember_string.vi"("Mode"=Remember_value_mode."Read and Write", "Input Value"=w807, "Ch name"=w809) -> ()  [unwired: 1 in, 8 out]
        n425 = local read "Port Name"() -> (w822:string)
        n426 = call "IFA300Command.vi"("Channel Name"="IFA300", "Port Name"=w822, "ValueToSet"=w814, "IFACommand"=w810, "Address"=w817) -> ("Error Description"=w821:string)  [unwired: 5 out]
      }
      frame "SquareWaveTest" {
        n427 = Unbundle By Name(w835) -> ("SquareWaveTest"=w830:bool)
        n428 = case shown="False" w830 {
          tunnel: [w838 w850] -> w831
          frame True {
            w842 = T1 "SqWaveVolts" ("IFA300Command")
            w846 = T1 "SqWaveFreq" ("IFA300Command")
            (unwired) T1 "SetHighpassFilter" ("IFA300Command")
            w843 = "IFA300" ("Channel Name")
            n429 = local read "Port Name"() -> (w844:string)
            n430 = call "SquareWaveDialog.vi"() -> ("FreqString"=w840:string, "VoltString"=w841:string)  [unwired: 8 in]
            n431 = call "Remember_string.vi"("Mode"=Remember_value_mode."Read and Write", "Input Value"=w840, "Ch name"=w846) -> ()  [unwired: 1 in, 8 out]
            n432 = call "IFA300Command.vi"("Channel Name"=w843, "Port Name"=w844, "ValueToSet"=w840, "IFACommand"=w846) -> ("Error Description"=w839:string)  [unwired: 1 in, 5 out]
            n433 = call "IFA300Command.vi"("Channel Name"=w843, "Port Name"=w844, "ValueToSet"=w841, "IFACommand"=w842) -> ("Error Description"=w837:string)  [unwired: 1 in, 5 out]
            n434 = call "Remember_string.vi"("Mode"=Remember_value_mode."Read and Write", "Input Value"=w841, "Ch name"=w842) -> ()  [unwired: 1 in, 8 out]
            n435 = Concatenate Strings(w839, w837) -> (w838:string)
          }
          frame False {
            w848 = "0"
            w852 = T1 "SqWaveVolts" ("IFA300Command")
            w856 = T1 "SqWaveFreq" ("IFA300Command")
            (unwired) T1 "SetHighpassFilter" ("IFA300Command")
            w853 = "IFA300" ("Channel Name")
            n436 = local read "Port Name"() -> (w854:string)
            n437 = call "Remember_string.vi"("Mode"=Remember_value_mode."Read and Write", "Input Value"=w848, "Ch name"=w856) -> ()  [unwired: 1 in, 8 out]
            n438 = call "IFA300Command.vi"("Channel Name"=w853, "Port Name"=w854, "ValueToSet"=w848, "IFACommand"=w856) -> ("Error Description"=w851:string)  [unwired: 1 in, 5 out]
            n439 = call "IFA300Command.vi"("Channel Name"=w853, "Port Name"=w854, "ValueToSet"=w848, "IFACommand"=w852) -> ("Error Description"=w849:string)  [unwired: 1 in, 5 out]
            n440 = call "Remember_string.vi"("Mode"=Remember_value_mode."Read and Write", "Input Value"=w848, "Ch name"=w852) -> ()  [unwired: 1 in, 8 out]
            n441 = Concatenate Strings(w851, w849) -> (w850:string)
          }
        }
        n442 = property on="SquareWaveTest" class="Bool (strict)"("Blinking"=w830) -> ()  [unwired: 2 in, 2 out]
        n443 = property on="RunAll" class="Bool (strict)"("Blinking"=w830) -> ()  [unwired: 2 in, 2 out]
        n444 = property on="StopAll" class="Bool (strict)"("Blinking"=w830) -> ()  [unwired: 2 in, 2 out]
      }
      frame "SetHotRes" {
        n445 = local read "Probe Resistance"() -> (w876:dbl)
        n446 = Unbundle By Name(w875) -> ("Channel Selector"=w866:string, "Overheat Setting"=w874:dbl)
        n447 = Multiply(x=w874, y=w876) -> (x*y=w864:dbl)
        n448 = local write "Hot Resistance"(w864) -> ()
        n449 = local read "Port Name"() -> (w873:string)
        n450 = Number To Fractional String(number=w864, precision (6)=i16 2) -> (F-format string=w870:string)  [unwired: 2 out]
        n451 = String Subset(string=w866, offset (0)=8) -> (substring=w867:string)  [unwired: 1 out]
        n452 = Decimal String To Number(string=w867) -> (number=w865:i32)  [unwired: 3 out]
        n453 = call "IFA300Command.vi"("Channel Name"="IFA300", "Port Name"=w873, "ValueToSet"=w870, "IFACommand"=T1 "SetHotResistance" ("IFA300Command"), "Address"=w865) -> ("Error Description"=w860:string)  [unwired: 5 out]
        n454 = Equal?(x=w860, y="") -> (x = y?=w861:bool)
        n455 = case shown="False" w861 {
          tunnel: w860 -> [w881 w885]
          tunnel: ["" ("Error Description") w885] -> w859
          frame False {
            n456 = Concatenate Strings("Unable to set Hot Res, check Cable Res and Cold Res values and retry." ("message"), "\n\n" ("string"), "Error Code: " ("string"), w881) -> (w880:string)
            n457 = One Button Dialog(message=w880) -> ()  [unwired: 2 out]
          }
          frame True {
          }
        }
      }
      frame "SetLowPassFilter" {
        w891 = T1 "SetLowpassFilter" ("IFA300Command")
        n458 = Unbundle By Name(w905) -> ("Channel Selector"=w888:string, "Low-Pass Filter"=w892:string)
        n459 = local read "ApplytoAll"() -> (w889:bool)
        n460 = case shown="True" w889 {
          tunnel: [w910 w912] -> w887
          tunnel: w888 -> [w910 _]
          tunnel: ["WriteFile" "HighPowerBridge"] -> w886
          frame False {
          }
          frame True {
            n461 = local read "CopytoChannels"() -> (w913:string[])
            n462 = Index Array(array=w913) -> (element=w912:string)  [unwired: 1 in]
          }
        }
        n463 = Equal?(x=w892, y="None") -> (x = y?=w899:bool)
        n464 = local read "Port Name"() -> (w906:string)
        n465 = Concatenate Strings(w888, "_" ("string"), w891) -> (w894:string)
        n466 = Select(t="BVSC", s=w899, f=w892) -> (s? t:f=w897:string)
        n467 = String Subset(string=w887, offset (0)=8) -> (substring=w903:string)  [unwired: 1 out]
        n468 = call "Remember_string.vi"("Mode"=Remember_value_mode."Read and Write", "Input Value"=w892, "Ch name"=w894) -> ()  [unwired: 1 in, 8 out]
        n469 = Decimal String To Number(string=w903) -> (number=w902:i32)  [unwired: 3 out]
        n470 = call "IFA300Command.vi"("Channel Name"="IFA300", "Port Name"=w906, "ValueToSet"=w897, "IFACommand"=w891, "Address"=w902) -> ("Error Description"=w901:string)  [unwired: 5 out]
      }
      frame "SetMode" {
        n471 = Unbundle By Name(w932) -> ("Channel Selector"=w928:string, "RunStandby"=w931:u8)
        n472 = String Subset(string=w928, offset (0)=8) -> (substring=w929:string)  [unwired: 1 out]
        n473 = Decimal String To Number(string=w929) -> (number=w927:i32)  [unwired: 3 out]
        n474 = case shown="0, Default" w931 {
          tunnel: [TRUE FALSE] -> w925
          tunnel: [FALSE TRUE] -> w917
          tunnel: w927 -> [w944 w951]
          tunnel: [w942 w949] -> w922
          frame 0, Default {
            n475 = local read "Port Name"() -> (w946:string)
            n476 = call "IFA300Command.vi"("Channel Name"="IFA300", "Port Name"=w946, "IFACommand"=T1 "StandbyMode" ("IFA300Command"), "Address"=w944) -> ("Error Description"=w942:string)  [unwired: 1 in, 5 out]
          }
          frame 1 {
            n477 = local read "Port Name"() -> (w953:string)
            n478 = call "IFA300Command.vi"("Channel Name"="IFA300", "Port Name"=w953, "IFACommand"=T1 "RunMode" ("IFA300Command"), "Address"=w951) -> ("Error Description"=w949:string)  [unwired: 1 in, 5 out]
          }
        }
        n479 = Decrement(x=w927) -> (x-1=w919:i32)
        n480 = Equal?(x=w922, y="") -> (x = y?=w923:bool)
        n481 = local write "Running"(w917) -> ()
        n482 = local write "Standby"(w925) -> ()
        n483 = case shown="False" w923 {
          tunnel: w922 -> [w936 w941]
          tunnel: ["" ("Error Description") w941] -> w921
          frame False {
            n484 = Concatenate Strings("Unable to set selected channel to Run mode.  Check Cable Res and Cold Res values and retry." ("message"), "\n\n" ("string"), "Error Code: " ("string"), w936) -> (w939:string)
            n485 = One Button Dialog(message=w939) -> ()  [unwired: 2 out]
          }
          frame True {
          }
        }
        n486 = local read "ModeArray"() -> (w920:cluster{bool, "Enable":bool}[])
        n487 = Bundle(w917, TRUE) -> (w916:cluster{bool, bool})  [unwired: 1 out]
        n488 = Replace Array Subset(array=w920, new element=w916, index=w919) -> (w918:cluster{bool, "Enable":bool}[])
        n489 = local write "ModeArray"(w918) -> ()
      }
      frame "SetOHRatio" {
        n490 = local read "ApplytoAll"() -> (w959:bool)
        n491 = Unbundle By Name(w967) -> ("Channel Selector"=w958:string, "Overheat Setting"=w966:dbl)
        n492 = case shown="True" w959 {
          tunnel: [w973 w980] -> w957
          tunnel: w958 -> [w973 _]
          tunnel: ["SetHotRes" w977] -> w956
          frame False {
          }
          frame True {
            n493 = local read "CopytoChannels"() -> (w981:string[])
            n494 = Delete From Array(array=w981) -> (deleted portion=w980:string, array with subset deleted=w979:string[])  [unwired: 2 in]
            n495 = Empty Array?(array=w979) -> (empty?=w975:bool)
            n496 = Not(x=w975) -> (.not. x?=w974:bool)
            n497 = local write "ApplytoAll"(w974) -> ()
            n498 = Select(t="Idle", s=w975, f="ApplytoAll") -> (s? t:f=w977:string)
          }
        }
        n499 = Number To Fractional String(number=w966, precision (6)=i16 1) -> (F-format string=w964:string)  [unwired: 2 out]
        n500 = Concatenate Strings(w957, "_" ("string"), T1 "OverrideOverheat" ("string")) -> (w962:string)
        n501 = call "Remember_string.vi"("Mode"=Remember_value_mode."Read and Write", "Input Value"=w964, "Ch name"=w962) -> ()  [unwired: 1 in, 8 out]
      }
      frame "SetOffset" {
        n502 = Unbundle By Name(w998) -> ("Channel Selector"=w984:string, "Offset"=w997:dbl)
        n503 = local read "ApplytoAll"() -> (w985:bool)
        n504 = case shown="True" w985 {
          tunnel: [w1001 w1003] -> w983
          tunnel: w984 -> [w1001 _]
          tunnel: ["ReadOffset" "SetHighPassFilter"] -> w982
          frame False {
          }
          frame True {
            n505 = local read "CopytoChannels"() -> (w1004:string[])
            n506 = Index Array(array=w1004) -> (element=w1003:string)  [unwired: 1 in]
          }
        }
        n507 = Number To Fractional String(number=w997, precision (6)=i16 2) -> (F-format string=w986:string)  [unwired: 2 out]
        n508 = String Subset(string=w983, offset (0)=8) -> (substring=w989:string)  [unwired: 1 out]
        n509 = Decimal String To Number(string=w989) -> (number=w988:i32)  [unwired: 3 out]
        n510 = local read "Port Name"() -> (w992:string)
        n511 = call "IFA300Command.vi"("Channel Name"="IFA300", "Port Name"=w992, "ValueToSet"=w986, "IFACommand"=T1 "SetOffset" ("IFA300Command"), "Address"=w988) -> ("Error Description"=w996:string)  [unwired: 5 out]
      }
      frame "SetProbeType" {
        n512 = Unbundle By Name(w1020) -> ("Channel Selector"=w1014:string, "Probe Type Selector"=w1019:u8)
        n513 = local read "ApplytoAll"() -> (w1015:bool)
        n514 = case shown="True" w1015 {
          tunnel: [w1026 w1028] -> w1005
          tunnel: w1014 -> [w1026 _]
          tunnel: ["WriteFile" "SetGain"] -> w1013
          frame False {
          }
          frame True {
            n515 = local read "CopytoChannels"() -> (w1029:string[])
            n516 = Index Array(array=w1029) -> (element=w1028:string)  [unwired: 1 in]
          }
        }
        n517 = String Subset(string=w1005, offset (0)=8) -> (substring=w1007:string)  [unwired: 1 out]
        n518 = case shown="0, Default" w1019 {
          tunnel: ["N" "F" "W"] -> w1009
          frame 0, Default {
          }
          frame 1 {
          }
          frame 2 {
          }
        }
        n519 = Decimal String To Number(string=w1007) -> (number=w1006:i32)  [unwired: 3 out]
        n520 = local read "Port Name"() -> (w1011:string)
        n521 = call "IFA300Command.vi"("Channel Name"="IFA300", "Port Name"=w1011, "ValueToSet"=w1009, "IFACommand"=T1 "SetProbeType" ("IFA300Command"), "Address"=w1006) -> ("Error Description"=w1018:string)  [unwired: 5 out]
      }
      frame "StandbyAll" {
        n522 = local read "Port Name"() -> (w1035:string)
        n523 = call "IFA300Command.vi"("Channel Name"="IFA300", "Port Name"=w1035, "IFACommand"=T1 "StandbyAll" ("IFA300Command")) -> ("Error Description"=w1033:string)  [unwired: 2 in, 5 out]
        n524 = local write "StopAll"(FALSE ("StopAll")) -> ()
      }
      frame "WriteFile" {
        w1072 = FALSE ("StopAll")
        w1049 = ""
        # "Running/Standby and Enable/Dissable into two arrays of strings."
        n525 = local read "Overheat (Running)"() -> (w1064:dbl)
        n526 = local read "TimeCableResMeas"() -> (w1062:string)
        n527 = local read "TimeCableResRead"() -> (w1061:string)
        n528 = local read "TimeColdResMeas"() -> (w1060:string)
        n529 = local read "TimeColdResRead"() -> (w1059:string)
        n530 = local read "Probe Resistance"() -> (w1066:dbl)
        n531 = local read "Cable Resistance"() -> (w1067:dbl)
        n532 = local read "Hot Resistance"() -> (w1065:dbl)
        n533 = local read "Temperature"() -> (w1070:dbl)
        n534 = local read "Port Name"() -> (w1063:string)
        n535 = for {
          tunnel: w1077 -> [w1221] mode=indexing
          shift-right: [w1217] -> w1057
          shift-left: w1049 -> [w1220]
          shift-right: [w1219] -> w1058
          shift-left: w1049 -> [w1218]
          n536 = Unbundle(w1221) -> (w1216:bool, "Enable"=w1214:bool)
          n537 = case shown="False" w1214 {
            tunnel: ["D" "E"] -> w1213
            frame False {
            }
            frame True {
            }
          }
          n538 = case shown="False" w1216 {
            tunnel: ["S" "R"] -> w1215
            frame False {
            }
            frame True {
            }
          }
          n539 = Concatenate Strings(w1220, w1215) -> (w1217:string)
          n540 = Concatenate Strings(w1218, w1213) -> (w1219:string)
        }
        n541 = local read "Running"() -> (w1069:bool)
        n542 = local read "Standby"() -> (w1068:bool)
        n543 = Bundle("Temperature"=w1070, "Running"=w1069, "Standby"=w1068, "Cable Resistance"=w1067, "Probe Resistance"=w1066, "Hot Resistance"=w1065, "Overheat (Running)"=w1064, "Port Name"=w1063, "TimeCableResMeas"=w1062, "TimeCableResRead"=w1061, "TimeColdResMeas"=w1060, "TimeColdResRead"=w1059) -> (w1054:T7)  [unwired: 1 out]
        n544 = Get Date/Time In Seconds() -> (seconds since 1Jan1904=w1076:timestamp)
        n545 = Format Date/Time String(seconds (now)=w1076) -> (date/time string=w1055:string)  [unwired: 2 out]
        n546 = To Double Precision Float(number=w1076) -> (double precision float=w1075:dbl)
        n547 = Number To Fractional String(number=w1075, precision (6)=i16 0) -> (F-format string=w1056:string)  [unwired: 2 out]
        n548 = call "IFA300HeaderList.vi"() -> ("appended array"=w1051:string[])  [unwired: 11 out]
        n549 = Bundle(cluster=T4 {"Running/Standby"="", "Enabled/Dissabled"="", "SecSince1904"="", "Date/TimeFileWritten"=""}, "Running/Standby"=w1057, "Enabled/Dissabled"=w1058, "SecSince1904"=w1056, "Date/TimeFileWritten"=w1055) -> (w1053:T4)
        n550 = for {
          tunnel: w1054 -> [w1085]
          tunnel: w1045 -> [w1084]
          tunnel: w1053 -> [w1086]
          tunnel: w1051 -> [w1083] mode=indexing
          tunnel: [w1082] -> w1050 mode=indexing
          n551 = case shown="\"Hot:Resistance\"" w1083 {
            tunnel: w1086 -> [_ _ _ w1099 _ _ _ _ _ _ _ _ _ _ _ _ _ _ _ _ _ _ _ _ w1181 _ w1188 _ _ _ _ _ _ _ w1212]
            tunnel: w1085 -> [_ w1095 _ _ _ _ _ _ w1117 _ _ _ _ _ w1138 _ w1144 w1148 _ _ _ _ _ _ _ w1184 _ w1191 _ w1202 w1204 w1206 w1208 w1210 _]
            tunnel: w1084 -> [w1089 _ w1097 _ w1102 w1106 w1108 w1111 _ w1119 w1122 w1127 _ w1134 _ w1142 _ _ w1151 w1157 w1161 w1167 w1172 w1177 _ _ _ _ w1196 _ _ _ _ _ _]
            tunnel: [w1087 w1092 w1096 w1098 w1101 w1105 w1107 w1109 w1115 w1118 w1121 w1126 "WriteFileError" ("Date/TimeFileWritten") w1132 w1136 w1140 w1143 w1146 w1149 w1156 w1162 w1165 w1170 w1175 w1180 w1182 w1187 w1189 w1194 w1200 w1203 w1205 w1207 w1209 w1211] -> w1082
            frame "Cable:Length:(m)" {
              n552 = Unbundle By Name(w1089) -> ("Cable Length"=w1088:u8)
              n553 = case shown="1" w1088 {
                tunnel: ["5" "30"] -> w1087
                frame 0, Default {
                }
                frame 1 {
                }
              }
            }
            frame "Cable:Resistance" {
              n554 = Unbundle By Name(w1095) -> ("Cable Resistance"=w1094:dbl)
              n555 = Number To Fractional String(number=w1094, precision (6)=i16 2) -> (F-format string=w1092:string)  [unwired: 2 out]
            }
            frame "Channel:Selector" {
              n556 = Unbundle By Name(w1097) -> ("Channel Selector"=w1096:string)
            }
            frame "Enabled/:Dissabled" {
              n557 = Unbundle By Name(w1099) -> ("Enabled/Dissabled"=w1098:string)
            }
            frame "End:Program" {
              n558 = Unbundle By Name(w1102) -> ("EndProgram"=w1100:bool)
              n559 = case shown="False" w1100 {
                tunnel: ["0" "1"] -> w1101
                frame False {
                }
                frame True {
                }
              }
            }
            frame "Gain" {
              n560 = Unbundle By Name(w1106) -> ("Gain"=w1105:string)
            }
            frame "High-Pass:Filter:(Hz)" {
              n561 = Unbundle By Name(w1108) -> ("High-Pass Filter"=w1107:string)
            }
            frame "High:Power:Bridge" {
              n562 = Unbundle By Name(w1111) -> ("High Power Bridge"=w1110:u8)
              n563 = case shown="1" w1110 {
                tunnel: ["Off" "On"] -> w1109
                frame 0, Default {
                }
                frame 1 {
                }
              }
            }
            frame "Hot:Resistance" {
              n564 = Unbundle By Name(w1117) -> ("Hot Resistance"=w1116:dbl)
              n565 = Number To Fractional String(number=w1116, precision (6)=i16 2) -> (F-format string=w1115:string)  [unwired: 2 out]
            }
            frame "Low-Pass:Filter:(Hz)" {
              n566 = Unbundle By Name(w1119) -> ("Low-Pass Filter"=w1118:string)
            }
            frame "Measure:Cable:Resistance" {
              n567 = Unbundle By Name(w1122) -> ("MeasCableRes"=w1120:bool)
              n568 = case shown="False" w1120 {
                tunnel: ["0" "1"] -> w1121
                frame False {
                }
                frame True {
                }
              }
            }
            frame "Measure:Probe:Resistance" {
              n569 = Unbundle By Name(w1127) -> ("MeasColdRes"=w1125:bool)
              n570 = case shown="False" w1125 {
                tunnel: ["0" "1"] -> w1126
                frame False {
                }
                frame True {
                }
              }
            }
            frame "NoMatch", Default {
            }
            frame "Offset" {
              n571 = Unbundle By Name(w1134) -> ("Offset"=w1133:dbl)
              n572 = Number To Fractional String(number=w1133, precision (6)=i16 2) -> (F-format string=w1132:string)  [unwired: 2 out]
            }
            frame "Overheat:(Measured)" {
              n573 = Unbundle By Name(w1138) -> ("Overheat (Running)"=w1137:dbl)
              n574 = Number To Fractional String(number=w1137, precision (6)=i16 1) -> (F-format string=w1136:string)  [unwired: 2 out]
            }
            frame "Overheat:Setting" {
              n575 = Unbundle By Name(w1142) -> ("Overheat Setting"=w1141:dbl)
              n576 = Number To Fractional String(number=w1141, precision (6)=i16 1) -> (F-format string=w1140:string)  [unwired: 2 out]
            }
            frame "Port:Name" {
              n577 = Unbundle By Name(w1144) -> ("Port Name"=w1143:string)
            }
            frame "Probe:Resistance" {
              n578 = Unbundle By Name(w1148) -> ("Probe Resistance"=w1147:dbl)
              n579 = Number To Fractional String(number=w1147, precision (6)=i16 2) -> (F-format string=w1146:string)  [unwired: 2 out]
            }
            frame "Probe:Type" {
              n580 = Unbundle By Name(w1151) -> ("Probe Type Selector"=w1150:u8)
              n581 = case shown="0, Default" w1150 {
                tunnel: ["Non-Cylindrical" "Film" "Wire"] -> w1149
                frame 0, Default {
                }
                frame 1 {
                }
                frame 2 {
                }
              }
            }
            frame "Read:Cable:Resistance" {
              n582 = Unbundle By Name(w1157) -> ("ReadCableRes"=w1155:bool)
              n583 = case shown="False" w1155 {
                tunnel: ["0" "1"] -> w1156
                frame False {
                }
                frame True {
                }
              }
            }
            frame "Read:Probe:Resistance" {
              n584 = Unbundle By Name(w1161) -> ("ReadColdRes"=w1160:bool)
              n585 = case shown="False" w1160 {
                tunnel: ["0" "1"] -> w1162
                frame False {
                }
                frame True {
                }
              }
            }
            frame "Reset" {
              n586 = Unbundle By Name(w1167) -> ("Reset IFA"=w1166:bool)
              n587 = case shown="False" w1166 {
                tunnel: ["0" "1"] -> w1165
                frame False {
                }
                frame True {
                }
              }
            }
            frame "Run:All" {
              n588 = Unbundle By Name(w1172) -> ("RunAll"=w1171:bool)
              n589 = case shown="False" w1171 {
                tunnel: ["0" "1"] -> w1170
                frame False {
                }
                frame True {
                }
              }
            }
            frame "Run:Standby:Switch" {
              n590 = Unbundle By Name(w1177) -> ("RunStandby"=w1176:u8)
              n591 = case shown="0, Default" w1176 {
                tunnel: ["Standby" "Run"] -> w1175
                frame 0, Default {
                }
                frame 1 {
                }
              }
            }
            frame "Running/:Standby" {
              n592 = Unbundle By Name(w1181) -> ("Running/Standby"=w1180:string)
            }
            frame "Running:Indicator" {
              n593 = Unbundle By Name(w1184) -> ("Running"=w1183:bool)
              n594 = case shown="False" w1183 {
                tunnel: ["0" "1"] -> w1182
                frame False {
                }
                frame True {
                }
              }
            }
            frame "Seconds:Since:1904" {
              n595 = Unbundle By Name(w1188) -> ("SecSince1904"=w1187:string)
            }
            frame "Standby:Indicator" {
              n596 = Unbundle By Name(w1191) -> ("Standby"=w1190:bool)
              n597 = case shown="False" w1190 {
                tunnel: ["0" "1"] -> w1189
                frame False {
                }
                frame True {
                }
              }
            }
            frame "Stop:All" {
              n598 = Unbundle By Name(w1196) -> ("StopAll"=w1195:bool)
              n599 = case shown="False" w1195 {
                tunnel: ["0" "1"] -> w1194
                frame False {
                }
                frame True {
                }
              }
            }
            frame "Temperature" {
              n600 = Unbundle By Name(w1202) -> ("Temperature"=w1201:dbl)
              n601 = Number To Fractional String(number=w1201, precision (6)=i16 2) -> (F-format string=w1200:string)  [unwired: 2 out]
            }
            frame "Time Cable:Resistance:Measured" {
              n602 = Unbundle By Name(w1204) -> ("TimeCableResMeas"=w1203:string)
            }
            frame "Time Cable:Resistance:Read" {
              n603 = Unbundle By Name(w1206) -> ("TimeCableResRead"=w1205:string)
            }
            frame "Time Probe:Resistance:Measured" {
              n604 = Unbundle By Name(w1208) -> ("TimeColdResMeas"=w1207:string)
            }
            frame "Time Probe:Resistance:Read" {
              n605 = Unbundle By Name(w1210) -> ("TimeColdResRead"=w1209:string)
            }
            frame "Time/Date:File:Written" {
              n606 = Unbundle By Name(w1212) -> ("Date/TimeFileWritten"=w1211:string)
            }
          }
        }
        n607 = Unbundle By Name(w1045) -> ("Channel Selector"=w1044:string, "Reset IFA"=w1040:bool)
        n608 = local read "EndProgram"() -> (w1047:bool)
        n609 = call "Write_out_serial_log.vi"("Header message"=w1044) -> ()
        n610 = Select(t="Initialize", s=w1040, f="Idle") -> (s? t:f=w1042:string)
        n611 = Bundle By Name(cluster=w1045, "RunAll"=w1072, "StopAll"=w1072, "MeasCableRes"=w1072, "ReadCableRes"=w1072, "MeasColdRes"=w1072, "ReadColdRes"=w1072, "Reset IFA"=w1072) -> (w1071:T5)
        n612 = Build Array(w1050) -> (w1073:string[][])
        n613 = Select(t="EndProgram", s=w1047, f=w1042) -> (s? t:f=w1048:string)
        n614 = call "WriteDatedLogFile.vi"("Channel Values"=w1073, "Channel names"=w1051, "LogFileName"="IFA300") -> ()  [unwired: 9 out]
      }
    }
    n615 = Equal?(x="", y=w8) -> (x = y?=w9:bool)
    n616 = case shown="False" w9 {
      tunnel: w8 -> [w18 _]
      frame False {
        n617 = One Button Dialog(message=w18) -> ()  [unwired: 2 out]
      }
      frame True {
      }
    }
    "Current Case" <- w12
  }
  n618 = local write "EndProgram"(w2) -> ()
